vi "EC_Applied_Motion_SXSYSZ_20170419A_3chNoBK_20190710.vi"() -> ()   [LabVIEW 2015]
uses:
  <vilib>/Instr/_visa.llb/VISA Configure Serial Port (Instr).vi
  <userlib>/caLab/Private/Put_DBL_PV.vi
  <userlib>/caLab/Private/Get_PV-1D.vi
  <userlib>/caLab/Private/Put_I32-1D_PV-1D.vi
  <userlib>/caLab/Private/Put_DBL-1D_PV-1D.vi
  <vilib>/Utility/file.llb/Write To Spreadsheet File (I64).vi
  <vilib>/Utility/file.llb/Read From Spreadsheet File (I64).vi
panel:
  out "Io":dbl
  out "APX:MZ_CHK":bool[](array[boolean])
  out "x .and. y?":bool
  out "element 7":u8
  out "Busy":bool
  out "element 6":bool
  out "element 5":bool
  out "element 4":bool
  out "element 3":bool
  out "element 2":bool
  out "element":bool
  out "status":u32
  in  "Local":bool=TRUE
  out "Move 5Z REQ":bool
  in  "Jog Z- CNTL":bool
  in  "Jog Z+ CNTL":bool
  in  "Jog Y- CNTL":bool
  in  "Jog Y+ CNTL":bool
  in  "Jog X- CNTL":bool
  in  "Jog X+ CNTL":bool
  out "APX:FZ_DOWN":u8
  out "APX:FZ_UP":u8
  out "APX:FY_DOWN":u8
  out "APX:FY_UP":u8
  out "APX:FX_DOWN":u8
  out "APX:FX_UP":u8
  out "FZ Jog Counts In Range?":bool
  out "FY Jog Counts In Range?":bool
  out "FX Jog Counts In Range?":bool
  in  "APX:MZ_CHK local":bool=TRUE
  out "Isolated from GND?":bool
  in  "Crash Override":bool
  out "Dev1 AI1":dbl
  in  "APX:FZabs":dbl
  in  "Move 5Z":bool
  out "APX:FZ_DOWN":bool
  out "APX:FX_DOWN":bool
  out "APX:FY_DOWN":bool
  out "Z Velocity MV mm/sec":dbl format="%.3f"
  out "Z Position MV mm":dbl=0.09994900000000001 format="%#_3g"
  out "Y Velocity MV mm/sec":dbl format="%.3f"
  out "Y Position MV mm":dbl=0.049996453999999996 format="%#_3g"
  out "X Velocity MV mm/sec":dbl format="%.3f"
  out "X Position MV mm":dbl=0.1000034915 format="%#_3g"
  in  "stop":bool
  in  "Tab Control 3":enum32{"Status", "Reset", "Error"}(tab)
  out "Y in Range":bool
  out "Y in Motion":bool
  out "X  in Range":bool
  out "X  in Motion":bool
  out "Z in Range":bool
  out "Z in Motion":bool
  out "X Ready":bool
  out "Y Ready":bool
  out "Z Ready":bool
  in  "Reset Y Position mm":dbl
  out "Reset Y Motor Steps":i32
  in  "Reset X Position mm":dbl
  out "Reset X Motor Steps":i32
  in  "Reset Z Position mm":dbl
  out "Reset Z Motor Steps":i32
  in  "Reset":bool
  out "error out":errorcluster
  in  "Tab Control":enum32{"mm", "Jog", "step", "info"}(tab)
  in  "APX:FXstep":dbl=0.1 min=0.1 max=0.2
  in  "FX Velocity SP mm/sec":dbl=0.010583500000000001
  in  "APX:FYstep":dbl=0.05 min=0.01 max=0.1
  in  "FY Velocity SP mm/sec":dbl=0.010583500000000001
  in  "APX:Fzstep":dbl=0.05 min=0.05 max=0.2
  in  "FZ Velocity SP mm/sec":dbl=0.0635
  in  "Z Jog Set":bool
  in  "Y Jog Set":bool
  in  "X Jog Set":bool
  in  "Reset Jog counts":bool
  in  "FZ Jog counts":i8
  in  "FY Jog counts":i8
  in  "FX Jog counts":i8
  out "FX Jog upper limit":dbl=40.0
  out "FX Jog lower limit":dbl=-40.0
  out "FY Jog lower limit":dbl=-15.0
  out "FY jog upper limit":dbl=15.0
  out "FZ jog upper limit":dbl=40.0
  out "FZ Jog lower limit":dbl=-40.0
  in  "X Velocity SP step/sec":i32 min=1 max=1000
  in  "Y Velocity SP step/sec":i32 min=1 max=1000
  in  "Z Velocity SP step/sec":i32 min=1 max=500
  in  "Y Step SP":i32=-20000 min=-800000 max=800000 step=500
  in  "X Step SP":i32=-20000 min=-750000 max=750000 step=500
  in  "Z Step SP":i32=-20000 min=-10240000 max=10240000 step=500
  out "X Step PV":i32 max=2000
  out "Y Step PV":i32 max=2000
  out "Z Step PV":i32 max=2000
  out "R Step PV":i32 max=2000
  out "X Run Current %":i32
  out "X Holding Current %":i32
  out "X velocity PV step/sec":i32
  out "X steps/rev":u32
  out "X mm/rev":dbl
  out "X offset mm":dbl
  out "X MINPOS":i32=-94296
  out "X MAXPOS":i32=-34296
  out "X COM PORT":refnum<visa-resource-name>="COM5"
  out "Y COM PORT":refnum<visa-resource-name>="COM5"
  out "Z COM PORT":refnum<visa-resource-name>="COM5"
  out "Y velocity PV step/sec":i32
  out "Y Run Current %":i32
  out "Y Holding Current %":i32
  out "Y MAXPOS":i32=-34296
  out "Y MINPOS":i32=-94296
  out "Y steps/rev":u32
  out "Y mm/rev":dbl
  out "Y offset mm":dbl
  out "Z  velocity PV step/sec":i32
  out "Z Run Current %":i32
  out "Z Holding Current %":i32
  out "Z MAXPOS":i32=-34296
  out "Z MINPOS":i32=-94296
  out "Z steps/rev":u32
  out "Z mm/rev":dbl
  out "Z offset mm":dbl
  out "APX:FZ_UP":bool
  out "Z Position mm PV":dbl format="%.3f"
  out "X Position mm PV":dbl format="%.3g"
  out "APX:FX_UP":bool
  out "Y Position mm PV":dbl format="%.3g"
  in  "Stop":bool
  out "APX:FY_UP":bool
  # "APX:FY"
  # "APX:FinePos"
  # "APX:FZ"
  # "x-ray"
  # "v20220620"
  # "APX:FX"
  # "SPEAR"
  # "Stage"
  # "Velovity"
  # "Jog step"
  # "Pos"
  # "sample to SSRL"
  # "FX"
  # "FY"
  # "FZ"
  # "These have to be positive"
  # "lim"
  # "connected"
  # "moving"
  # "R,L = green"
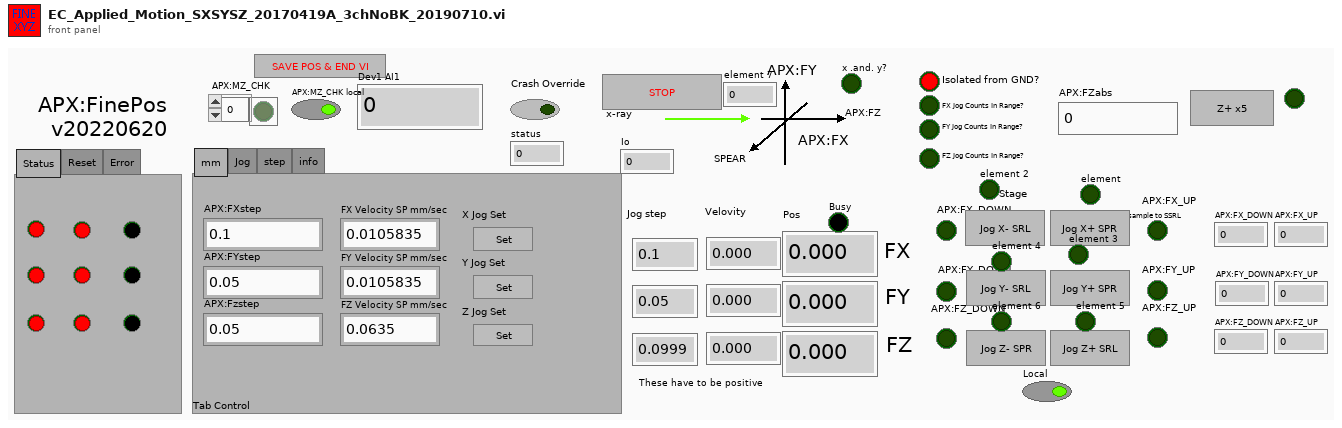
[diagram p1: front panel]
types:
  T1 = cluster{"first row[0]":i64, "first row[1]":i64, "first row[2]":i64, "first row[3]":i64, "first row[4]":i64, "first row[5]":i64, "first row[6]":i64, "first row[7]":i64, "first row[8]":i64}
  T2 = enum16{"Power-up Signature", "Accel Rate", "Accel Max", "Bit Rate", "Buffer Status", "Change Current", "Commence Jogging", "Change Jog Speed", "Continue", "Define Address", "Distance for FC,FM,FO,FY", "Decel Rate", "Distance or Position", "Define Limits", "Encoder Deadband", "Encoder Function", "Encoder Position", "Encoder Ratio", "Feed to Length with Speed Change", "Feed to Length", "Feed to Sensor with Mask Dist", "Feed to Length & Set Output", "Feed to Position", "Feed to Sensor", "Feed to Sensor w/safety", "Follow Handwheel", "Immediate Distance?", "Immediate Encoder?", "Immediate Low Output", "Immediate High Output", "Immediate Position?", "Input Status?", "Jog Accel/Decel", "Jog Disable", "Jog Enable", "Jog Speed", "Motor Disable", "Motor Enable", "Microstep Resolution", "Power up Current", "Power up Mode", "Pause", "Request Status", "Revision Level?", "Seek Home", "Stop Jogging", "Stop & Kill Buffer", "Set Output", "Set ABS Position", "Send String", "Stop", "Velocity for Speed Change", "Velocity Setting", "Wait for Input", "Wait Time"}
  T3 = enum8{"Enabled", "Disabled", "Disabled and Grayed Out"}
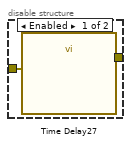
[diagram p7: hidden frame]
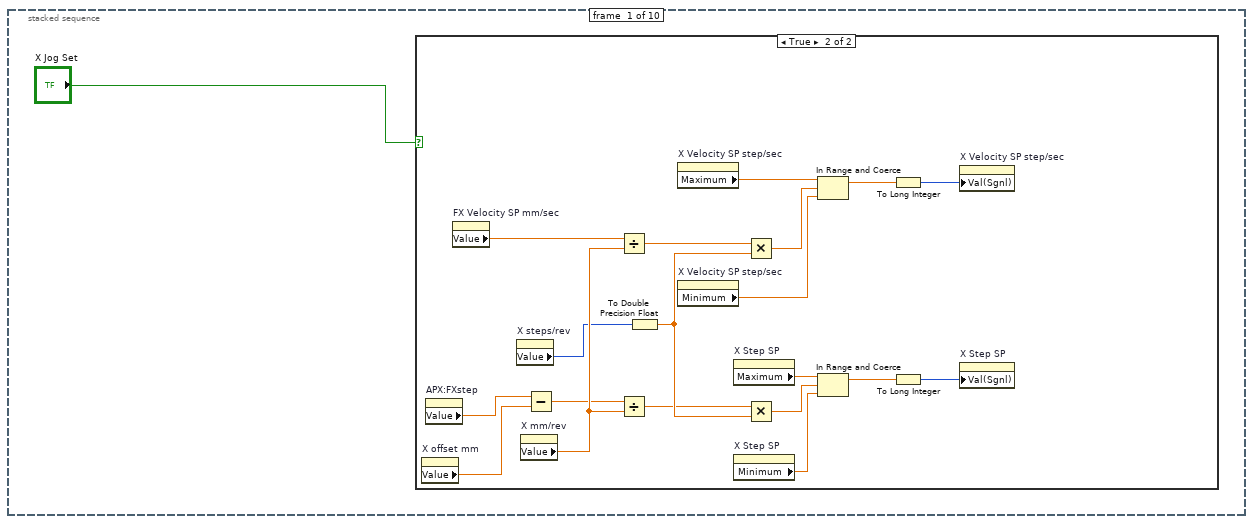
[diagram p9: hidden frame]
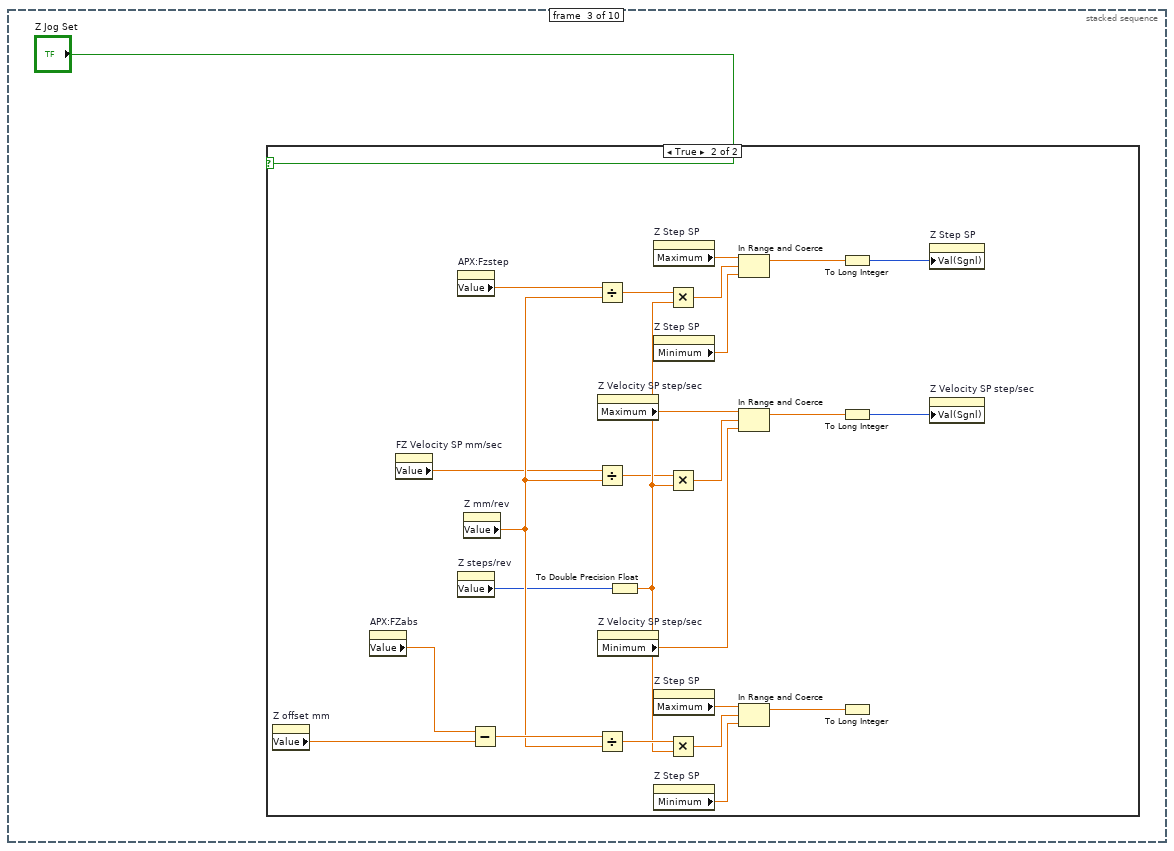
[diagram p12: hidden frame]
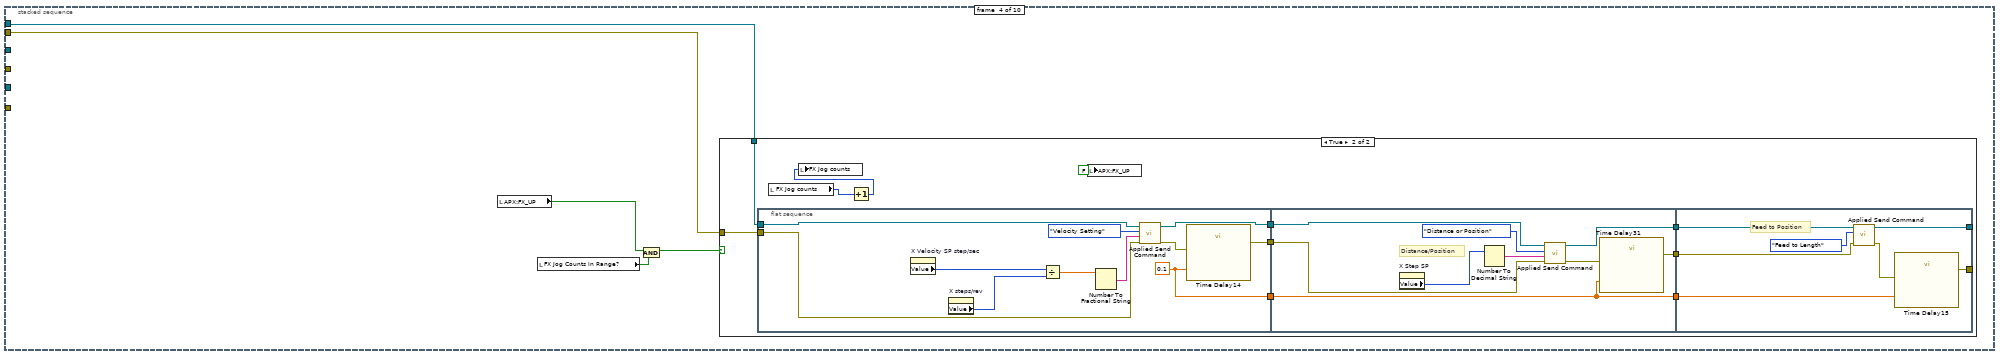
[diagram p14: hidden frame]
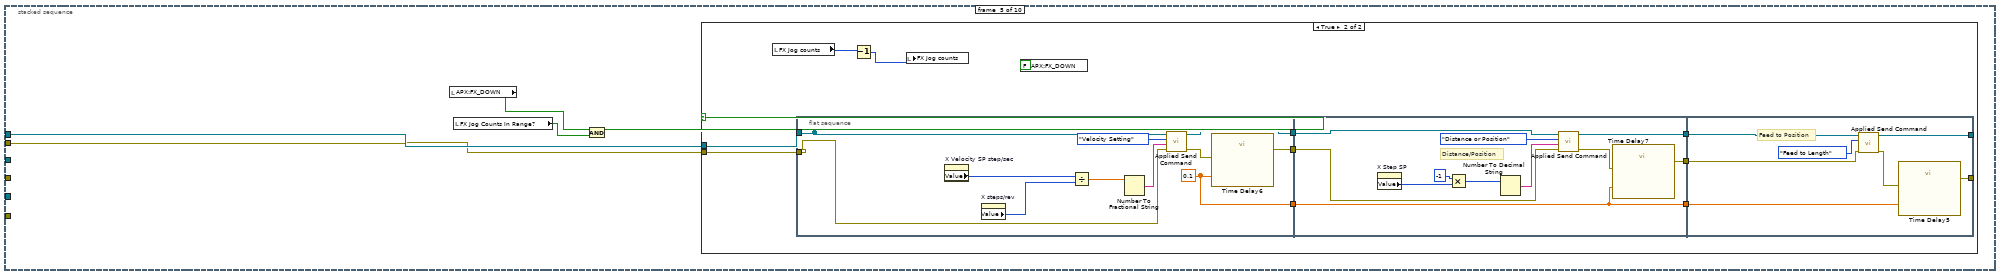
[diagram p16: hidden frame]
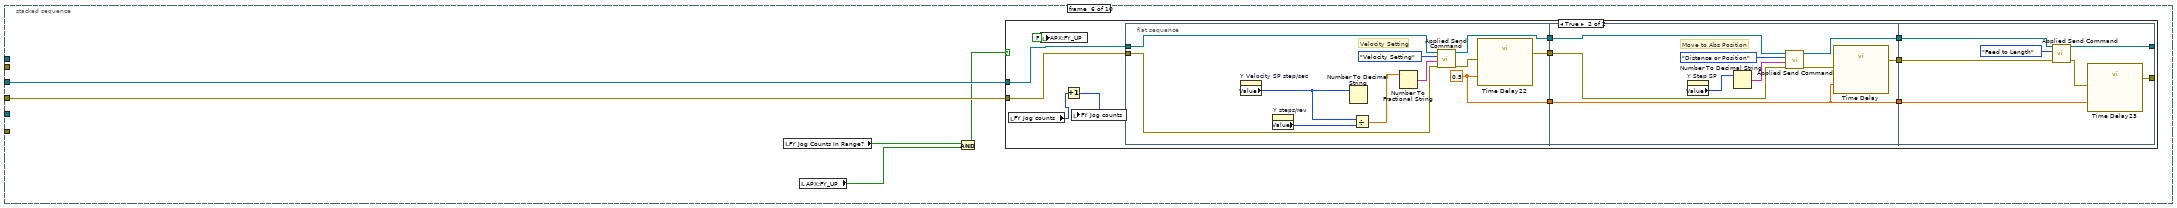
[diagram p18: hidden frame]
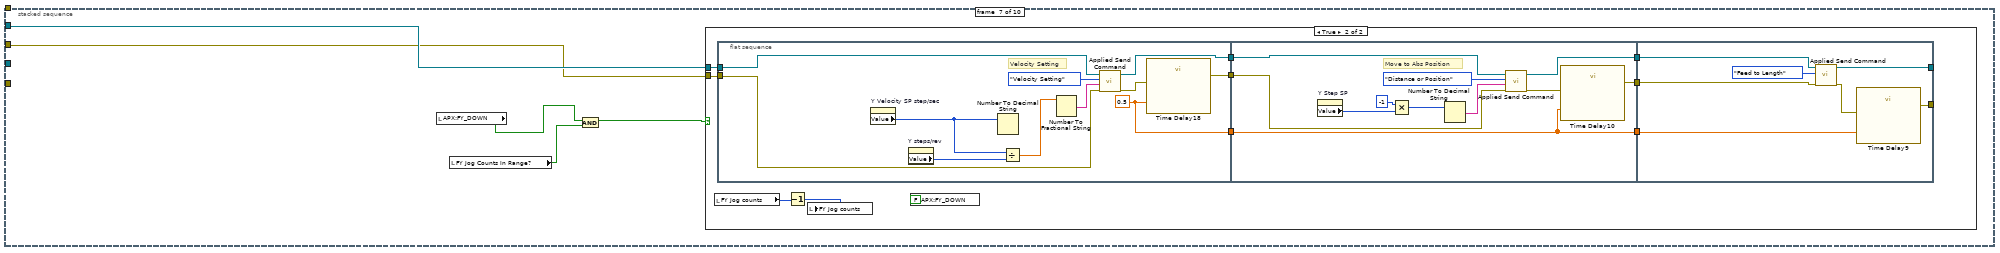
[diagram p20: hidden frame]
diagram:
  n1 = disable-structure shown="Disabled" {
    frame Disabled {
      (unwired) FALSE
      n2 = flat-sequence {
        frame #0 {
        }
        frame #1 {
          n3 = call-poly <vilib>:"Read From Spreadsheet File.vi"("file path (dialog if empty)"=path "S:/SSE/SCL2/POS.TXT") -> ("first row"=w43:i64[])  [unwired: 6 in, 4 out]
          n4 = Array To Cluster(array=w43) -> (cluster=w44:T1)
          n5 = Unbundle(w44) -> ("first row[0]"=w46:i64, "first row[1]"=w47:i64, "first row[2]"=w48:i64)  [unwired: 6 out]
          n6 = property on="Reset X Motor Steps" class="DigNum (strict)"("Val(Sgnl)"=w46) -> ()  [unwired: 2 in, 2 out]
          n7 = property on="Reset Y Motor Steps" class="DigNum (strict)"("Val(Sgnl)"=w47) -> ()  [unwired: 2 in, 2 out]
          n8 = property on="Reset Z Motor Steps" class="DigNum (strict)"("Val(Sgnl)"=w48) -> ()  [unwired: 2 in, 2 out]
        }
      }
    }
    frame Enabled {
    }
  }
  n9 = flat-sequence {
    tunnel: [w65] -> w18
    tunnel: [w64] -> w17
    tunnel: w18 -> [w82]
    tunnel: w17 -> [w81]
    tunnel: [w80] -> w16
    tunnel: [w79] -> w15
    tunnel: [w86] -> w40
    tunnel: w16 -> [w94]
    tunnel: w15 -> [w93]
    tunnel: [w87] -> w14
    tunnel: w40 -> [w108]
    tunnel: [w107] -> w34
    tunnel: [w105] -> w33
    tunnel: [w110] -> w32
    tunnel: w14 -> [w109]
    tunnel: [w116] -> w38
    tunnel: [w117] -> w39
    tunnel: w34 -> [w117]
    tunnel: w33 -> [w116]
    tunnel: w32 -> [w115]
    frame #0 {
      "X Run Current %" <- 100 ("Run Current %")
      "X Holding Current %" <- 50 ("Holding Current %")
    }
    frame #1 {
      w51 = T3."Enabled" ("Disabled")
      n10 = property on="APX:FX_UP" class="Bool"("DisabledEnum"=w51) -> ()  [unwired: 2 in, 2 out]
      n11 = property on="APX:FX_DOWN" class="Bool"("DisabledEnum"=w51) -> ()  [unwired: 2 in, 2 out]
      n12 = property on="APX:FY_UP" class="Bool"("DisabledEnum"=w51) -> ()  [unwired: 2 in, 2 out]
      n13 = property on="APX:FZ_UP" class="Bool"("DisabledEnum"=w51) -> ()  [unwired: 2 in, 2 out]
      n14 = property on="APX:FY_DOWN" class="Bool"("DisabledEnum"=w51) -> ()  [unwired: 2 in, 2 out]
      n15 = property on="APX:FZ_DOWN" class="Bool"("DisabledEnum"=w51) -> ()  [unwired: 2 in, 2 out]
    }
    frame #2 {
      w54 = 0.21167 ("MM/rev")
      w57 = u32 20000 ("step/rev")
      w52 = 1000 ("Value (Signaling)")
      (unwired) 0.01 ("Value (Signaling)")
      n16 = property on="X Velocity SP step/sec" class="DigNum (strict)"("Minimum"=1.0 ("Data Entry Limits:Minimum")) -> ()  [unwired: 2 in, 2 out]
      n17 = property on="X Velocity SP step/sec" class="DigNum (strict)"("Val(Sgnl)"=w52) -> ()  [unwired: 2 in, 2 out]
      n18 = To Double Precision Float(number=w57) -> (double precision float=w56:dbl)
      n19 = To Double Precision Float(number=w52) -> (double precision float=w58:dbl)
      n20 = property on="X Velocity SP step/sec" class="DigNum (strict)"("Maximum"=w58) -> ()  [unwired: 2 in, 2 out]
      n21 = Divide(x=w58, y=w56) -> (x/y=w53:dbl)
      n22 = Multiply(x=w53, y=w54) -> (x*y=w55:dbl)
      n23 = property on="FX Velocity SP mm/sec" class="DigNum (strict)"("Val(Sgnl)"=w55) -> ()  [unwired: 2 in, 2 out]
      "X steps/rev" <- w57
      "X mm/rev" <- w54
    }
    frame #3 {
      w63 = -750000 ("lower limit")
      w62 = 750000 ("upper limit")
      n24 = local write "X Step SP"(9449 ("X Step SP")) -> ()
      n25 = property on="X Step SP" class="DigNum (strict)"("Maximum"=w62) -> ()  [unwired: 2 in, 2 out]
      n26 = property on="X Step SP" class="DigNum (strict)"("Minimum"=w63) -> ()  [unwired: 2 in, 2 out]
      "X offset mm" <- 0.0 ("offset")
      "X MAXPOS" <- w62
      "X MINPOS" <- w63
    }
    frame #4 {
      w72 = refnum<visa-resource-name> "COM21" ("COM PORT")
      w70 = u16 0 items=["None", "XON/XOFF", "RTS/CTS", "XON/XOFF & RTS/CTS", "DTR/DSR", "XON/XOFF & DTR/DSR"] ("flow control (0:none)")
      w69 = u16 10 items=["1.0"=10, "1.5"=15, "2.0"=20] ("stop bits (10: 1 bit)")
      # "Stop bits"
      n27 = call-poly "VISA Configure Serial Port"("VISA resource name"=w72, "timeout (10sec)"=u32 10000, "baud rate (9600)"=u32 9600, "data bits (8)"=u16 8, "parity (0:none)"=enum16{"None", "Odd", "Even", "Mark", "Space"}."None", "stop bits (10: 1 bit)"=w69, "flow control (0:none)"=w70) -> ("VISA resource name out"=w65:refnum<visa-resource-name>, "error out"=w64:errorcluster)  [unwired: 7 in]
      "X COM PORT" <- w72
    }
    frame #5 {
      n28 = property on="X Run Current" class="DigNum (strict)"() -> ("Value"=w77:i32)  [unwired: 2 in, 2 out]
      n29 = Divide(x=w77, y=100) -> (x/y=w74:dbl)
      n30 = Multiply(x=3.5 ("y"), y=w74) -> (x*y=w76:dbl)
      n31 = Number To Fractional String(number=w76) -> (F-format string=w78:string)  [unwired: 3 in]
      n32 = call "Applied Send Command.vi"("error in (no error)"=w81, "Extra"=w78, "Command"=T2."Change Current", "VISA resource name"=w82) -> ("error out"=w80:errorcluster, "VISA resource name out"=w79:refnum<visa-resource-name>)  [unwired: 3 in, 1 out]
    }
    frame #6 {
      # "VELOCITY"
      n33 = property on="X Velocity SP step/sec" class="DigNum (strict)"() -> ("Value"=w90:i32)  [unwired: 2 in, 2 out]
      n34 = property on="X steps/rev" class="DigNum (strict)"() -> ("Value"=w89:u32)  [unwired: 2 in, 2 out]
      n35 = Divide(x=w90, y=w89) -> (x/y=w88:dbl)
      n36 = Absolute Value(x=w88) -> (abs(x)=w84:dbl)
      n37 = Number To Fractional String(number=w84) -> (F-format string=w95:string)  [unwired: 3 in]
      n38 = call "Applied Send Command.vi"("error in (no error)"=w94, "Extra"=w95, "Command"=T2."Velocity Setting", "VISA resource name"=w93) -> ("error out"=w96:errorcluster, "VISA resource name out"=w103:refnum<visa-resource-name>)  [unwired: 3 in, 1 out]
      n39 = call "Time Delay30"("error in (no error)"=w96, "Delay Time (s)"=0.1) -> ("error out"=w101:errorcluster)  [unwired: 9 in]
      n40 = call "Applied Send Command.vi"("error in (no error)"=w101, "Extra"="", "Command"=T2."Velocity Setting", "VISA resource name"=w103) -> ("error out"=w86:errorcluster, "read buffer"=w99:string, "VISA resource name out"=w87:refnum<visa-resource-name>)  [unwired: 3 in]
      n41 = Fract/Exp String To Number(string=w99, offset=3) -> (number=w92:dbl)  [unwired: 2 in, 1 out]
      n42 = Multiply(x=w92, y=w89) -> (x*y=w91:dbl)
      n43 = property on="X velocity PV step/sec" class="DigNum (strict)"("Val(Sgnl)"=w91) -> ()  [unwired: 2 in, 2 out]
    }
    frame #7 {
      # "GET CURRENT POSITION"
      n44 = call "Applied Send Command.vi"("error in (no error)"=w108, "Extra"="", "Command"=T2."Immediate Position?", "VISA resource name"=w109) -> ("error out"=w106:errorcluster, "read buffer"=w112:string, "VISA resource name out"=w107:refnum<visa-resource-name>)  [unwired: 3 in]
      n45 = call "Time Delay13"("error in (no error)"=w106, "Delay Time (s)"=0.1) -> ("error out"=w105:errorcluster)  [unwired: 9 in]
      n46 = Hexadecimal String To Number(string=w112, offset=3) -> (number=w110:u32)  [unwired: 1 in, 1 out]
    }
    frame #8 {
      n47 = disable-structure shown="Disabled" {
        disable-tunnel: w115 -> [w118 _]
        frame Disabled {
          n48 = property on="X Step SP" class="DigNum (strict)"("Val(Sgnl)"=w118) -> ()  [unwired: 2 in, 2 out]
          n49 = property on="X Step SP" class="DigNum (strict)"() -> ("Maximum"=w121:dbl)  [unwired: 2 in, 2 out]
          n50 = property on="X Step SP" class="DigNum (strict)"() -> ("Minimum"=w120:dbl)  [unwired: 2 in, 2 out]
          n51 = In Range and Coerce(upper limit=w121, x=w118, lower limit=w120) -> (In Range?=w119:bool)  [unwired: 1 out]
          n52 = property on="X  in Range" class="Bool (strict)"("Val(Sgnl)"=w119) -> ()  [unwired: 2 in, 2 out]
        }
        frame Enabled {
        }
      }
    }
  }
  n53 = flat-sequence {
    tunnel: [w137] -> w5
    tunnel: [w136] -> w4
    tunnel: w5 -> [w151]
    tunnel: w4 -> [w150]
    tunnel: [w149] -> w3
    tunnel: [w148] -> w2
    tunnel: [w160] -> w31
    tunnel: [w159] -> w30
    tunnel: w3 -> [w162]
    tunnel: w2 -> [w161]
    tunnel: w31 -> [w177]
    tunnel: w30 -> [w176]
    tunnel: [w178] -> w29
    tunnel: [w179] -> w28
    tunnel: [w180] -> w1
    tunnel: [w190] -> w26
    tunnel: [w191] -> w27
    tunnel: w29 -> [w191]
    tunnel: w28 -> [w190]
    tunnel: w1 -> [w189]
    frame #0 {
      "Z Run Current %" <- 100 ("Z Run Current %")
      "Z Holding Current %" <- 50 ("Z Holding Current %")
    }
    frame #1 {
    }
    frame #2 {
      (unwired) 0.05 ("Value (Signaling)")
      w126 = 2.54 ("Z mm/rev")
      w125 = u32 20000 ("step/rev")
      w127 = 500 ("Value (Signaling)")
      n54 = property on="Z Velocity SP step/sec" class="DigNum (strict)"("Minimum"=1.0 ("Data Entry Limits:Minimum")) -> ()  [unwired: 2 in, 2 out]
      n55 = property on="Z Velocity SP step/sec" class="DigNum (strict)"("Val(Sgnl)"=w127) -> ()  [unwired: 2 in, 2 out]
      n56 = To Double Precision Float(number=w125) -> (double precision float=w130:dbl)
      n57 = To Double Precision Float(number=w127) -> (double precision float=w131:dbl)
      n58 = property on="Z Velocity SP step/sec" class="DigNum (strict)"("Maximum"=w131) -> ()  [unwired: 2 in, 2 out]
      n59 = Divide(x=w131, y=w130) -> (x/y=w128:dbl)
      n60 = Multiply(x=w128, y=w126) -> (x*y=w129:dbl)
      n61 = property on="FZ Velocity SP mm/sec" class="DigNum (strict)"("Val(Sgnl)"=w129) -> ()  [unwired: 2 in, 2 out]
      "Z mm/rev" <- w126
      "Z steps/rev" <- w125
    }
    frame #3 {
      w134 = -10240000 ("lower limit")
      w133 = 10240000 ("upper limit")
      n62 = property on="Z Step SP" class="DigNum (strict)"("Minimum"=w134) -> ()  [unwired: 2 in, 2 out]
      n63 = local write "Z Step SP"(394 ("Z Step SP")) -> ()
      n64 = property on="Z Step SP" class="DigNum (strict)"("Maximum"=w133) -> ()  [unwired: 2 in, 2 out]
      "Z offset mm" <- 0.0 ("Z offset mm")
      "Z MINPOS" <- w134
      "Z MAXPOS" <- w133
    }
    frame #4 {
      w144 = refnum<visa-resource-name> "COM23" ("COM PORT")
      w142 = u16 0 items=["None", "XON/XOFF", "RTS/CTS", "XON/XOFF & RTS/CTS", "DTR/DSR", "XON/XOFF & DTR/DSR"] ("flow control (0:none)")
      w141 = u16 10 items=["1.0"=10, "1.5"=15, "2.0"=20] ("stop bits (10: 1 bit)")
      # "Stop bits"
      n65 = call-poly "VISA Configure Serial Port"("VISA resource name"=w144, "timeout (10sec)"=u32 10000, "baud rate (9600)"=u32 9600, "data bits (8)"=u16 8, "parity (0:none)"=enum16{"None", "Odd", "Even", "Mark", "Space"}."None", "stop bits (10: 1 bit)"=w141, "flow control (0:none)"=w142) -> ("VISA resource name out"=w137:refnum<visa-resource-name>, "error out"=w136:errorcluster)  [unwired: 7 in]
      "Z COM PORT" <- w144
    }
    frame #5 {
      # "Run Current %"
      n66 = property on="Z Run Current %" class="DigNum (strict)"() -> ("Value"=w152:i32)  [unwired: 2 in, 2 out]
      n67 = Divide(x=w152, y=100) -> (x/y=w153:dbl)
      n68 = Multiply(x=w153, y=3.5) -> (x*y=w147:dbl)
      n69 = Number To Fractional String(number=w147) -> (F-format string=w154:string)  [unwired: 3 in]
      n70 = call "Applied Send Command.vi"("error in (no error)"=w150, "Extra"=w154, "Command"=T2."Change Current", "VISA resource name"=w151) -> ("error out"=w148:errorcluster, "VISA resource name out"=w149:refnum<visa-resource-name>)  [unwired: 3 in, 1 out]
    }
    frame #6 {
      # "VELOCITY"
      n71 = property on="Z Velocity SP step/sec" class="DigNum (strict)"() -> ("Value"=w157:i32)  [unwired: 2 in, 2 out]
      n72 = property on="Z steps/rev" class="DigNum (strict)"() -> ("Value"=w158:u32)  [unwired: 2 in, 2 out]
      n73 = Divide(x=w157, y=w158) -> (x/y=w165:dbl)
      n74 = Absolute Value(x=w165) -> (abs(x)=w156:dbl)
      n75 = Number To Fractional String(number=w156) -> (F-format string=w167:string)  [unwired: 3 in]
      n76 = call "Applied Send Command.vi"("error in (no error)"=w161, "Extra"=w167, "Command"=T2."Velocity Setting", "VISA resource name"=w162) -> ("error out"=w168:errorcluster, "VISA resource name out"=w175:refnum<visa-resource-name>)  [unwired: 3 in, 1 out]
      n77 = call "Time Delay2"("error in (no error)"=w168, "Delay Time (s)"=0.1) -> ("error out"=w173:errorcluster)  [unwired: 9 in]
      n78 = call "Applied Send Command.vi"("error in (no error)"=w173, "Extra"="", "Command"=T2."Velocity Setting", "VISA resource name"=w175) -> ("error out"=w159:errorcluster, "read buffer"=w171:string, "VISA resource name out"=w160:refnum<visa-resource-name>)  [unwired: 3 in]
      n79 = Fract/Exp String To Number(string=w171, offset=3) -> (number=w166:dbl)  [unwired: 2 in, 1 out]
      n80 = Multiply(x=w166, y=w158) -> (x*y=w163:dbl)
      n81 = property on="Z  velocity PV step/sec" class="DigNum (strict)"("Val(Sgnl)"=w163) -> ()  [unwired: 2 in, 2 out]
    }
    frame #7 {
      # "GET CURRENT POSITION"
      n82 = call "Applied Send Command.vi"("error in (no error)"=w176, "Extra"="", "Command"=T2."Immediate Position?", "VISA resource name"=w177) -> ("error out"=w182:errorcluster, "read buffer"=w184:string, "VISA resource name out"=w178:refnum<visa-resource-name>)  [unwired: 3 in]
      n83 = call "Time Delay8"("error in (no error)"=w182, "Delay Time (s)"=0.1) -> ("error out"=w179:errorcluster)  [unwired: 9 in]
      n84 = Hexadecimal String To Number(string=w184, offset=3) -> (number=w180:u32)  [unwired: 1 in, 1 out]
    }
    frame #8 {
      n85 = disable-structure shown="Disabled" {
        disable-tunnel: w189 -> [w194 _]
        frame Disabled {
          n86 = property on="Z Step SP" class="DigNum (strict)"("Val(Sgnl)"=w194) -> ()  [unwired: 2 in, 2 out]
          n87 = property on="Z Step SP" class="DigNum (strict)"() -> ("Maximum"=w193:dbl)  [unwired: 2 in, 2 out]
          n88 = property on="Z Step SP" class="DigNum (strict)"() -> ("Minimum"=w192:dbl)  [unwired: 2 in, 2 out]
          n89 = In Range and Coerce(upper limit=w193, x=w194, lower limit=w192) -> (In Range?=w195:bool)  [unwired: 1 out]
          n90 = property on="Z in Range" class="Bool (strict)"("Val(Sgnl)"=w195) -> ()  [unwired: 2 in, 2 out]
        }
        frame Enabled {
        }
      }
      n91 = property on="Z Position MV mm" class="DigNum (strict)"("Val(Sgnl)"=0.05 ("Value (Signaling)")) -> ()  [unwired: 2 in, 2 out]
      n92 = property on="X Position MV mm" class="DigNum (strict)"("Val(Sgnl)"=0.1 ("Value (Signaling)")) -> ()  [unwired: 2 in, 2 out]
    }
  }
  n93 = flat-sequence {
    tunnel: [w211] -> w13
    tunnel: [w210] -> w12
    tunnel: w13 -> [w225]
    tunnel: w12 -> [w224]
    tunnel: [w223] -> w11
    tunnel: [w222] -> w10
    tunnel: w11 -> [w234]
    tunnel: w10 -> [w233]
    tunnel: [w232] -> w9
    tunnel: [w231] -> w8
    tunnel: [w251] -> w35
    tunnel: w9 -> [w254]
    tunnel: w8 -> [w253]
    tunnel: [w252] -> w7
    tunnel: [w250] -> w6
    tunnel: [w262] -> w41
    tunnel: [w264] -> w42
    tunnel: w35 -> [w262]
    tunnel: w7 -> [w264]
    tunnel: w6 -> [w263]
    frame #0 {
      "Y Run Current %" <- 100 ("Run Current %")
      "Y Holding Current %" <- 50 ("Holding Current %")
    }
    frame #1 {
    }
    frame #2 {
      w200 = 0.21167 ("MM/rev")
      w203 = u32 20000 ("step/rev")
      w198 = 1000 ("Value (Signaling)")
      (unwired) 0.01 ("Value (Signaling)")
      n94 = property on="Y Velocity SP step/sec" class="DigNum (strict)"("Minimum"=1.0 ("Data Entry Limits:Minimum")) -> ()  [unwired: 2 in, 2 out]
      n95 = property on="Y Velocity SP step/sec" class="DigNum (strict)"("Val(Sgnl)"=w198) -> ()  [unwired: 2 in, 2 out]
      n96 = To Double Precision Float(number=w203) -> (double precision float=w202:dbl)
      n97 = To Double Precision Float(number=w198) -> (double precision float=w204:dbl)
      n98 = property on="Y Velocity SP step/sec" class="DigNum (strict)"("Maximum"=w204) -> ()  [unwired: 2 in, 2 out]
      n99 = Divide(x=w204, y=w202) -> (x/y=w199:dbl)
      n100 = Multiply(x=w199, y=w200) -> (x*y=w201:dbl)
      n101 = property on="FY Velocity SP mm/sec" class="DigNum (strict)"("Val(Sgnl)"=w201) -> ()  [unwired: 2 in, 2 out]
      "Y steps/rev" <- w203
      "Y mm/rev" <- w200
    }
    frame #3 {
      w208 = -800000 ("lower limit")
      w209 = 800000 ("upper limit")
      n102 = local write "Y Step SP"(4724 ("Y Step SP")) -> ()
      n103 = property on="Y Step SP" class="DigNum (strict)"("Maximum"=w209) -> ()  [unwired: 2 in, 2 out]
      n104 = property on="Y Step SP" class="DigNum (strict)"("Minimum"=w208) -> ()  [unwired: 2 in, 2 out]
      "Y MAXPOS" <- w209
      "Y MINPOS" <- w208
      "Y offset mm" <- 0.0 ("offset")
    }
    frame #4 {
      w218 = refnum<visa-resource-name> "COM22" ("COM PORT")
      w216 = u16 0 items=["None", "XON/XOFF", "RTS/CTS", "XON/XOFF & RTS/CTS", "DTR/DSR", "XON/XOFF & DTR/DSR"] ("flow control (0:none)")
      w215 = u16 10 items=["1.0"=10, "1.5"=15, "2.0"=20] ("stop bits (10: 1 bit)")
      # "Stop bits"
      n105 = call-poly "VISA Configure Serial Port"("VISA resource name"=w218, "timeout (10sec)"=u32 10000, "baud rate (9600)"=u32 9600, "data bits (8)"=u16 8, "parity (0:none)"=enum16{"None", "Odd", "Even", "Mark", "Space"}."None", "stop bits (10: 1 bit)"=w215, "flow control (0:none)"=w216) -> ("VISA resource name out"=w211:refnum<visa-resource-name>, "error out"=w210:errorcluster)  [unwired: 7 in]
      "Y COM PORT" <- w218
    }
    frame #5 {
      n106 = property on="Y Run Current %" class="DigNum (strict)"() -> ("Value"=w226:i32)  [unwired: 2 in, 2 out]
      n107 = Divide(x=w226, y=100) -> (x/y=w227:dbl)
      n108 = Multiply(x=w227, y=3.5) -> (x*y=w221:dbl)
      n109 = Number To Fractional String(number=w221) -> (F-format string=w228:string)  [unwired: 3 in]
      n110 = call "Applied Send Command.vi"("error in (no error)"=w224, "Extra"=w228, "Command"=T2."Change Current", "VISA resource name"=w225) -> ("error out"=w222:errorcluster, "VISA resource name out"=w223:refnum<visa-resource-name>)  [unwired: 3 in, 1 out]
    }
    frame #6 {
      # "VELOCITY"
      n111 = property on="Y Velocity SP step/sec" class="DigNum (strict)"() -> ("Value"=w235:i32)  [unwired: 2 in, 2 out]
      n112 = property on="Y steps/rev" class="DigNum (strict)"() -> ("Value"=w238:u32)  [unwired: 2 in, 2 out]
      n113 = Divide(x=w235, y=w238) -> (x/y=w237:dbl)
      n114 = Absolute Value(x=w237) -> (abs(x)=w230:dbl)
      n115 = Number To Fractional String(number=w230) -> (F-format string=w241:string)  [unwired: 3 in]
      n116 = call "Applied Send Command.vi"("error in (no error)"=w233, "Extra"=w241, "Command"=T2."Velocity Setting", "VISA resource name"=w234) -> ("error out"=w242:errorcluster, "VISA resource name out"=w249:refnum<visa-resource-name>)  [unwired: 3 in, 1 out]
      n117 = call "Time Delay36"("error in (no error)"=w242, "Delay Time (s)"=0.1) -> ("error out"=w247:errorcluster)  [unwired: 9 in]
      n118 = call "Applied Send Command.vi"("error in (no error)"=w247, "Extra"="", "Command"=T2."Velocity Setting", "VISA resource name"=w249) -> ("error out"=w231:errorcluster, "read buffer"=w245:string, "VISA resource name out"=w232:refnum<visa-resource-name>)  [unwired: 3 in]
      n119 = Fract/Exp String To Number(string=w245, offset=3) -> (number=w240:dbl)  [unwired: 2 in, 1 out]
      n120 = Multiply(x=w240, y=w238) -> (x*y=w239:dbl)
      n121 = property on="Y velocity PV step/sec" class="DigNum (strict)"("Val(Sgnl)"=w239) -> ()  [unwired: 2 in, 2 out]
    }
    frame #7 {
      # "GET CURRENT POSITION"
      n122 = call "Applied Send Command.vi"("error in (no error)"=w253, "Extra"="", "Command"=T2."Immediate Position?", "VISA resource name"=w254) -> ("error out"=w256:errorcluster, "read buffer"=w258:string, "VISA resource name out"=w252:refnum<visa-resource-name>)  [unwired: 3 in]
      n123 = call "Time Delay37"("error in (no error)"=w256, "Delay Time (s)"=0.1) -> ("error out"=w251:errorcluster)  [unwired: 9 in]
      n124 = Hexadecimal String To Number(string=w258, offset=3) -> (number=w250:u32)  [unwired: 1 in, 1 out]
    }
    frame #8 {
      n125 = disable-structure shown="Disabled" {
        disable-tunnel: w263 -> [w267 _]
        frame Disabled {
          n126 = property on="Y Step SP" class="DigNum (strict)"("Val(Sgnl)"=w267) -> ()  [unwired: 2 in, 2 out]
          n127 = property on="Y Step SP" class="DigNum (strict)"() -> ("Maximum"=w266:dbl)  [unwired: 2 in, 2 out]
          n128 = property on="Y Step SP" class="DigNum (strict)"() -> ("Minimum"=w265:dbl)  [unwired: 2 in, 2 out]
          n129 = In Range and Coerce(upper limit=w266, x=w267, lower limit=w265) -> (In Range?=w268:bool)  [unwired: 1 out]
          n130 = property on="Y in Range" class="Bool (strict)"("Val(Sgnl)"=w268) -> ()  [unwired: 2 in, 2 out]
        }
        frame Enabled {
        }
      }
      n131 = property on="Y Position MV mm" class="DigNum (strict)"("Val(Sgnl)"=0.05 ("Value (Signaling)")) -> ()  [unwired: 2 in, 2 out]
    }
  }
  n132 = while {
    tunnel: w42 -> [w273]
    tunnel: w41 -> [w272]
    tunnel: [w285] -> w22
    tunnel: [w284] -> w23
    tunnel: w39 -> [w275]
    tunnel: w38 -> [w274]
    tunnel: [w282] -> w37
    tunnel: [w281] -> w36
    tunnel: w27 -> [w271]
    tunnel: w26 -> [w270]
    tunnel: [w280] -> w25
    tunnel: [w279] -> w24
    tunnel: [w278] -> _
    tunnel: [w277] -> _
    stop <- "stop" stop-if-true
    n133 = flat-sequence {
      frame #0 {
      }
      frame #1 {
      }
    }
    n134 = flat-sequence {
      frame #0 {
      }
      frame #1 {
      }
    }
    n135 = flat-sequence {
      frame #0 {
        n136 = local read "X Position mm PV"() -> (w292:dbl)
        n137 = local read "Z Position mm PV"() -> (w293:dbl)
        n138 = local read "Y Position mm PV"() -> (w291:dbl)
        n139 = Build Array(w292, w291, w293) -> (w286:dbl[])
        n140 = Build Array("APX:PiezeX", "APX:PiezeY", "APX:PiezeZ") -> (w287:string[])
        n141 = call-poly <userlib>:"CaLabPut.vi"("Values"=w286, "PV Names"=w287) -> ()  [unwired: 6 in, 4 out]
      }
    }
    n142 = flat-sequence {
      frame #0 {
        w297 = -40.0 ("lower limit")
        w296 = 40.0 ("upper limit")
        w301 = -15.0 ("lower limit")
        w300 = 15.0 ("upper limit")
        w305 = -40.0 ("lower limit")
        w304 = 40.0 ("upper limit")
        n143 = local read "FZ Jog counts"() -> (w295:i8)
        n144 = local read "FY Jog counts"() -> (w299:i8)
        n145 = local read "FX Jog counts"() -> (w303:i8)
        n146 = In Range and Coerce(upper limit=w304, x=w303, lower limit=w305) -> (In Range?=→"FX Jog Counts In Range?":bool)  [unwired: 1 out]
        n147 = In Range and Coerce(upper limit=w300, x=w299, lower limit=w301) -> (In Range?=→"FY Jog Counts In Range?":bool)  [unwired: 1 out]
        n148 = In Range and Coerce(upper limit=w296, x=w295, lower limit=w297) -> (In Range?=→"FZ Jog Counts In Range?":bool)  [unwired: 1 out]
        "FX Jog upper limit" <- w304
        "FX Jog lower limit" <- w305
        "FY jog upper limit" <- w300
        "FY Jog lower limit" <- w301
        "FZ jog upper limit" <- w296
        "FZ Jog lower limit" <- w297
      }
    }
    n149 = stacked-sequence {
      tunnel: w275 -> [_ _ _ w477 w520 _ _ _ _ _]
      tunnel: w274 -> [_ _ _ w476 w519 _ _ _ _ _]
      tunnel: w273 -> [_ _ _ _ _ w565 w608 _ _ _]
      tunnel: w272 -> [_ _ _ _ _ w564 w607 _ _ _]
      tunnel: w271 -> [_ _ _ _ _ _ _ w653 w696 w740]
      tunnel: w270 -> [_ _ _ _ _ _ _ w652 w695 w741]
      frame #0 {
        n150 = case shown="True" "X Jog Set" {
          frame False {
          }
          frame True {
            n151 = property on="X offset mm" class="DigNum (strict)"() -> ("Value"=w412:dbl)  [unwired: 2 in, 2 out]
            n152 = property on="APX:FXstep" class="DigNum (strict)"() -> ("Value"=w413:dbl)  [unwired: 2 in, 2 out]
            n153 = property on="FX Velocity SP mm/sec" class="DigNum (strict)"() -> ("Value"=w419:dbl)  [unwired: 2 in, 2 out]
            n154 = property on="X steps/rev" class="DigNum (strict)"() -> ("Value"=w410:u32)  [unwired: 2 in, 2 out]
            n155 = property on="X mm/rev" class="DigNum (strict)"() -> ("Value"=w426:dbl)  [unwired: 2 in, 2 out]
            n156 = Subtract(x=w413, y=w412) -> (x-y=w409:dbl)
            n157 = Divide(x=w419, y=w426) -> (x/y=w418:dbl)
            n158 = Divide(x=w409, y=w426) -> (x/y=w408:dbl)
            n159 = To Double Precision Float(number=w410) -> (double precision float=w425:dbl)
            n160 = property on="X Velocity SP step/sec" class="DigNum (strict)"() -> ("Maximum"=w423:dbl)  [unwired: 2 in, 2 out]
            n161 = property on="X Velocity SP step/sec" class="DigNum (strict)"() -> ("Minimum"=w424:dbl)  [unwired: 2 in, 2 out]
            n162 = property on="X Step SP" class="DigNum (strict)"() -> ("Maximum"=w416:dbl)  [unwired: 2 in, 2 out]
            n163 = property on="X Step SP" class="DigNum (strict)"() -> ("Minimum"=w417:dbl)  [unwired: 2 in, 2 out]
            n164 = Multiply(x=w418, y=w425) -> (x*y=w421:dbl)
            n165 = Multiply(x=w408, y=w425) -> (x*y=w414:dbl)
            n166 = In Range and Coerce(upper limit=w423, x=w421, lower limit=w424) -> (coerced(x)=w422:dbl)  [unwired: 1 out]
            n167 = In Range and Coerce(upper limit=w416, x=w414, lower limit=w417) -> (coerced(x)=w415:dbl)  [unwired: 1 out]
            n168 = To Long Integer(number=w422) -> (32bit integer=w420:i32)
            n169 = To Long Integer(number=w415) -> (32bit integer=w411:i32)
            n170 = property on="X Velocity SP step/sec" class="DigNum (strict)"("Val(Sgnl)"=w420) -> ()  [unwired: 2 in, 2 out]
            n171 = property on="X Step SP" class="DigNum (strict)"("Val(Sgnl)"=w411) -> ()  [unwired: 2 in, 2 out]
          }
        }
      }
      frame #1 {
        n172 = case shown="True" "Y Jog Set" {
          frame False {
          }
          frame True {
            n173 = property on="Y offset mm" class="DigNum (strict)"() -> ("Value"=w432:dbl)  [unwired: 2 in, 2 out]
            n174 = property on="APX:FYstep" class="DigNum (strict)"() -> ("Value"=w433:dbl)  [unwired: 2 in, 2 out]
            n175 = property on="FY Velocity SP mm/sec" class="DigNum (strict)"() -> ("Value"=w439:dbl)  [unwired: 2 in, 2 out]
            n176 = property on="Y steps/rev" class="DigNum (strict)"() -> ("Value"=w430:u32)  [unwired: 2 in, 2 out]
            n177 = property on="Y mm/rev" class="DigNum (strict)"() -> ("Value"=w446:dbl)  [unwired: 2 in, 2 out]
            n178 = Subtract(x=w433, y=w432) -> (x-y=w429:dbl)
            n179 = Divide(x=w439, y=w446) -> (x/y=w438:dbl)
            n180 = Divide(x=w429, y=w446) -> (x/y=w428:dbl)
            n181 = To Double Precision Float(number=w430) -> (double precision float=w445:dbl)
            n182 = property on="Y Velocity SP step/sec" class="DigNum (strict)"() -> ("Maximum"=w443:dbl)  [unwired: 2 in, 2 out]
            n183 = property on="Y Velocity SP step/sec" class="DigNum (strict)"() -> ("Minimum"=w444:dbl)  [unwired: 2 in, 2 out]
            n184 = property on="Y Step SP" class="DigNum (strict)"() -> ("Maximum"=w436:dbl)  [unwired: 2 in, 2 out]
            n185 = property on="Y Step SP" class="DigNum (strict)"() -> ("Minimum"=w437:dbl)  [unwired: 2 in, 2 out]
            n186 = Multiply(x=w438, y=w445) -> (x*y=w441:dbl)
            n187 = Multiply(x=w428, y=w445) -> (x*y=w434:dbl)
            n188 = In Range and Coerce(upper limit=w443, x=w441, lower limit=w444) -> (coerced(x)=w442:dbl)  [unwired: 1 out]
            n189 = In Range and Coerce(upper limit=w436, x=w434, lower limit=w437) -> (coerced(x)=w435:dbl)  [unwired: 1 out]
            n190 = To Long Integer(number=w442) -> (32bit integer=w440:i32)
            n191 = To Long Integer(number=w435) -> (32bit integer=w431:i32)
            n192 = property on="Y Velocity SP step/sec" class="DigNum (strict)"("Val(Sgnl)"=w440) -> ()  [unwired: 2 in, 2 out]
            n193 = property on="Y Step SP" class="DigNum (strict)"("Val(Sgnl)"=w431) -> ()  [unwired: 2 in, 2 out]
          }
        }
      }
      frame #2 {
        n194 = case shown="True" "Z Jog Set" {
          frame False {
          }
          frame True {
            n195 = property on="Z offset mm" class="DigNum (strict)"() -> ("Value"=w470:dbl)  [unwired: 2 in, 2 out]
            n196 = property on="APX:FZabs" class="DigNum (strict)"() -> ("Value"=w472:dbl)  [unwired: 2 in, 2 out]
            n197 = property on="FZ Velocity SP mm/sec" class="DigNum (strict)"() -> ("Value"=w457:dbl)  [unwired: 2 in, 2 out]
            n198 = property on="APX:Fzstep" class="DigNum (strict)"() -> ("Value"=w451:dbl)  [unwired: 2 in, 2 out]
            n199 = property on="Z steps/rev" class="DigNum (strict)"() -> ("Value"=w449:u32)  [unwired: 2 in, 2 out]
            n200 = property on="Z mm/rev" class="DigNum (strict)"() -> ("Value"=w469:dbl)  [unwired: 2 in, 2 out]
            n201 = Subtract(x=w472, y=w470) -> (x-y=w471:dbl)
            n202 = Divide(x=w451, y=w469) -> (x/y=w448:dbl)
            n203 = Divide(x=w457, y=w469) -> (x/y=w456:dbl)
            n204 = Divide(x=w471, y=w469) -> (x/y=w468:dbl)
            n205 = property on="Z Velocity SP step/sec" class="DigNum (strict)"() -> ("Maximum"=w461:dbl)  [unwired: 2 in, 2 out]
            n206 = property on="Z Velocity SP step/sec" class="DigNum (strict)"() -> ("Minimum"=w462:dbl)  [unwired: 2 in, 2 out]
            n207 = To Double Precision Float(number=w449) -> (double precision float=w467:dbl)
            n208 = property on="Z Step SP" class="DigNum (strict)"() -> ("Maximum"=w454:dbl)  [unwired: 2 in, 2 out]
            n209 = property on="Z Step SP" class="DigNum (strict)"() -> ("Minimum"=w455:dbl)  [unwired: 2 in, 2 out]
            n210 = property on="Z Step SP" class="DigNum (strict)"() -> ("Maximum"=w464:dbl)  [unwired: 2 in, 2 out]
            n211 = property on="Z Step SP" class="DigNum (strict)"() -> ("Minimum"=w465:dbl)  [unwired: 2 in, 2 out]
            n212 = Multiply(x=w448, y=w467) -> (x*y=w452:dbl)
            n213 = Multiply(x=w456, y=w467) -> (x*y=w459:dbl)
            n214 = Multiply(x=w468, y=w467) -> (x*y=w466:dbl)
            n215 = In Range and Coerce(upper limit=w454, x=w452, lower limit=w455) -> (coerced(x)=w453:dbl)  [unwired: 1 out]
            n216 = In Range and Coerce(upper limit=w461, x=w459, lower limit=w462) -> (coerced(x)=w460:dbl)  [unwired: 1 out]
            n217 = In Range and Coerce(upper limit=w464, x=w466, lower limit=w465) -> (coerced(x)=w463:dbl)  [unwired: 1 out]
            n218 = To Long Integer(number=w453) -> (32bit integer=w450:i32)
            n219 = To Long Integer(number=w460) -> (32bit integer=w458:i32)
            n220 = To Long Integer(number=w463) -> ()  [unwired: 1 out]
            n221 = property on="Z Step SP" class="DigNum (strict)"("Val(Sgnl)"=w450) -> ()  [unwired: 2 in, 2 out]
            n222 = property on="Z Velocity SP step/sec" class="DigNum (strict)"("Val(Sgnl)"=w458) -> ()  [unwired: 2 in, 2 out]
          }
        }
      }
      frame #3 {
        n223 = local read "APX:FX_UP"() -> (w473:bool)
        n224 = local read "FX Jog Counts In Range?"() -> (w474:bool)
        n225 = And(x=w473, y=w474) -> (x .and. y?=w475:bool)
        n226 = case shown="True" w475 {
          tunnel: w477 -> [_ w482]
          tunnel: w476 -> [_ w481]
          frame False {
          }
          frame True {
            n227 = flat-sequence {
              tunnel: [w493] -> w488
              tunnel: [w490] -> w487
              tunnel: [w489] -> w486
              tunnel: w482 -> [w495]
              tunnel: w481 -> [w494]
              tunnel: w488 -> [w502]
              tunnel: [w501] -> w485
              tunnel: w487 -> [w503]
              tunnel: [w504] -> w484
              tunnel: w486 -> [w500]
              tunnel: [w500] -> w483
              tunnel: w485 -> [w515]
              tunnel: w484 -> [w514]
              tunnel: [w513] -> _
              tunnel: [w512] -> _
              tunnel: w483 -> [w511]
              frame #0 {
                w489 = 0.1 ("Delay Time (s)")
                n228 = property on="X Velocity SP step/sec" class="DigNum (strict)"() -> ("Value"=w492:i32)  [unwired: 2 in, 2 out]
                n229 = property on="X steps/rev" class="DigNum (strict)"() -> ("Value"=w496:u32)  [unwired: 2 in, 2 out]
                n230 = Divide(x=w492, y=w496) -> (x/y=w497:dbl)
                n231 = Number To Fractional String(number=w497) -> (F-format string=w498:string)  [unwired: 3 in]
                n232 = call "Applied Send Command.vi"("error in (no error)"=w494, "Extra"=w498, "Command"=T2."Velocity Setting", "VISA resource name"=w495) -> ("error out"=w491:errorcluster, "VISA resource name out"=w493:refnum<visa-resource-name>)  [unwired: 3 in, 1 out]
                n233 = call "Time Delay14"("error in (no error)"=w491, "Delay Time (s)"=w489) -> ("error out"=w490:errorcluster)  [unwired: 9 in]
              }
              frame #1 {
                # "Distance/Position"
                n234 = property on="X Step SP" class="DigNum (strict)"() -> ("Value"=w505:i32)  [unwired: 2 in, 2 out]
                n235 = Number To Decimal String(number=w505) -> (decimal integer string=w507:string)  [unwired: 1 in]
                n236 = call "Applied Send Command.vi"("error in (no error)"=w503, "Extra"=w507, "Command"=T2."Distance or Position", "VISA resource name"=w502) -> ("error out"=w506:errorcluster, "VISA resource name out"=w501:refnum<visa-resource-name>)  [unwired: 3 in, 1 out]
                n237 = call "Time Delay31"("error in (no error)"=w506, "Delay Time (s)"=w500) -> ("error out"=w504:errorcluster)  [unwired: 9 in]
              }
              frame #2 {
                # "Feed to Position"
                n238 = call "Applied Send Command.vi"("error in (no error)"=w514, "Command"=T2."Feed to Length", "VISA resource name"=w515) -> ("error out"=w509:errorcluster, "VISA resource name out"=w513:refnum<visa-resource-name>)  [unwired: 4 in, 1 out]
                n239 = call "Time Delay15"("error in (no error)"=w509, "Delay Time (s)"=w511) -> ("error out"=w512:errorcluster)  [unwired: 9 in]
              }
            }
            n240 = local read "FX Jog counts"() -> (w480:i8)
            n241 = Increment(x=w480) -> (x+1=w479:i8)
            n242 = local write "FX Jog counts"(w479) -> ()
            n243 = local write "APX:FX_UP"(FALSE ("Jog X+")) -> ()
          }
        }
      }
      frame #4 {
        n244 = local read "APX:FX_DOWN"() -> (w516:bool)
        n245 = local read "FX Jog Counts In Range?"() -> (w517:bool)
        n246 = And(x=w516, y=w517) -> (x .and. y?=w518:bool)
        n247 = case shown="True" w518 {
          tunnel: w520 -> [_ w525]
          tunnel: w519 -> [_ w524]
          frame False {
          }
          frame True {
            n248 = local read "FX Jog counts"() -> (w523:i8)
            n249 = flat-sequence {
              tunnel: [w538] -> w531
              tunnel: [w535] -> w530
              tunnel: [w534] -> w529
              tunnel: [w533] -> _
              tunnel: w525 -> [w533]
              tunnel: w524 -> [w532]
              tunnel: w531 -> [w547]
              tunnel: [w546] -> w528
              tunnel: w530 -> [w548]
              tunnel: [w549] -> w527
              tunnel: w529 -> [w545]
              tunnel: [w545] -> w526
              tunnel: w528 -> [w560]
              tunnel: w527 -> [w559]
              tunnel: [w558] -> _
              tunnel: [w557] -> _
              tunnel: w526 -> [w556]
              frame #0 {
                w534 = 0.1 ("Delay Time (s)")
                n250 = property on="X Velocity SP step/sec" class="DigNum (strict)"() -> ("Value"=w537:i32)  [unwired: 2 in, 2 out]
                n251 = property on="X steps/rev" class="DigNum (strict)"() -> ("Value"=w539:u32)  [unwired: 2 in, 2 out]
                n252 = Divide(x=w537, y=w539) -> (x/y=w540:dbl)
                n253 = Number To Fractional String(number=w540) -> (F-format string=w541:string)  [unwired: 3 in]
                n254 = call "Applied Send Command.vi"("error in (no error)"=w532, "Extra"=w541, "Command"=T2."Velocity Setting", "VISA resource name"=w533) -> ("error out"=w536:errorcluster, "VISA resource name out"=w538:refnum<visa-resource-name>)  [unwired: 3 in, 1 out]
                n255 = call "Time Delay6"("error in (no error)"=w536, "Delay Time (s)"=w534) -> ("error out"=w535:errorcluster)  [unwired: 9 in]
              }
              frame #1 {
                # "Distance/Position"
                n256 = property on="X Step SP" class="DigNum (strict)"() -> ("Value"=w550:i32)  [unwired: 2 in, 2 out]
                n257 = Multiply(x=-1, y=w550) -> (x*y=w544:i32)
                n258 = Number To Decimal String(number=w544) -> (decimal integer string=w552:string)  [unwired: 1 in]
                n259 = call "Applied Send Command.vi"("error in (no error)"=w548, "Extra"=w552, "Command"=T2."Distance or Position", "VISA resource name"=w547) -> ("error out"=w551:errorcluster, "VISA resource name out"=w546:refnum<visa-resource-name>)  [unwired: 3 in, 1 out]
                n260 = call "Time Delay7"("error in (no error)"=w551, "Delay Time (s)"=w545) -> ("error out"=w549:errorcluster)  [unwired: 9 in]
              }
              frame #2 {
                # "Feed to Position"
                n261 = call "Applied Send Command.vi"("error in (no error)"=w559, "Command"=T2."Feed to Length", "VISA resource name"=w560) -> ("error out"=w554:errorcluster, "VISA resource name out"=w558:refnum<visa-resource-name>)  [unwired: 4 in, 1 out]
                n262 = call "Time Delay5"("error in (no error)"=w554, "Delay Time (s)"=w556) -> ("error out"=w557:errorcluster)  [unwired: 9 in]
              }
            }
            n263 = Decrement(x=w523) -> (x-1=w522:i8)
            n264 = local write "FX Jog counts"(w522) -> ()
            n265 = local write "APX:FX_DOWN"(FALSE ("Jog X-")) -> ()
          }
        }
      }
      frame #5 {
        n266 = local read "FY Jog Counts In Range?"() -> (w562:bool)
        n267 = local read "APX:FY_UP"() -> (w561:bool)
        n268 = And(x=w562, y=w561) -> (x .and. y?=w563:bool)
        n269 = case shown="True" w563 {
          tunnel: w565 -> [_ w570]
          tunnel: w564 -> [_ w569]
          frame False {
          }
          frame True {
            n270 = local read "FY Jog counts"() -> (w568:i8)
            n271 = local write "APX:FY_UP"(FALSE ("Jog Y+")) -> ()
            n272 = Increment(x=w568) -> (x+1=w567:i8)
            n273 = local write "FY Jog counts"(w567) -> ()
            n274 = flat-sequence {
              tunnel: [w583] -> w576
              tunnel: [w578] -> w575
              tunnel: [w577] -> w574
              tunnel: w569 -> [w582]
              tunnel: w570 -> [w581]
              tunnel: [w594] -> w573
              tunnel: [w589] -> w572
              tunnel: w576 -> [w592]
              tunnel: w575 -> [w593]
              tunnel: w574 -> [w590]
              tunnel: [w590] -> w571
              tunnel: [w599] -> _
              tunnel: [w602] -> _
              tunnel: w573 -> [w601]
              tunnel: w572 -> [w600]
              tunnel: w571 -> [w603]
              frame #0 {
                w577 = 0.5 ("Delay Time (s)")
                # "Velocity Setting"
                n275 = property on="Y Velocity SP step/sec" class="DigNum (strict)"() -> ("Value"=w586:i32)  [unwired: 2 in, 2 out]
                n276 = property on="Y steps/rev" class="DigNum (strict)"() -> ("Value"=w585:u32)  [unwired: 2 in, 2 out]
                n277 = Number To Decimal String(number=w586) -> ()  [unwired: 1 in, 1 out]
                n278 = Divide(x=w586, y=w585) -> (x/y=w587:dbl)
                n279 = Number To Fractional String(number=w587) -> (F-format string=w580:string)  [unwired: 3 in]
                n280 = call "Applied Send Command.vi"("error in (no error)"=w582, "Extra"=w580, "Command"=T2."Velocity Setting", "VISA resource name"=w581) -> ("error out"=w579:errorcluster, "VISA resource name out"=w583:refnum<visa-resource-name>)  [unwired: 3 in, 1 out]
                n281 = call "Time Delay22"("error in (no error)"=w579, "Delay Time (s)"=w577) -> ("error out"=w578:errorcluster)  [unwired: 9 in]
              }
              frame #1 {
                # "Move to Abs Position"
                n282 = property on="Y Step SP" class="DigNum (strict)"() -> ("Value"=w596:i32)  [unwired: 2 in, 2 out]
                n283 = Number To Decimal String(number=w596) -> (decimal integer string=w591:string)  [unwired: 1 in]
                n284 = call "Applied Send Command.vi"("error in (no error)"=w593, "Extra"=w591, "Command"=T2."Distance or Position", "VISA resource name"=w592) -> ("error out"=w588:errorcluster, "VISA resource name out"=w594:refnum<visa-resource-name>)  [unwired: 3 in, 1 out]
                n285 = call "Time Delay"("error in (no error)"=w588, "Delay Time (s)"=w590) -> ("error out"=w589:errorcluster)  [unwired: 9 in]
              }
              frame #2 {
                n286 = call "Applied Send Command.vi"("error in (no error)"=w600, "Command"=T2."Feed to Length", "VISA resource name"=w601) -> ("error out"=w597:errorcluster, "VISA resource name out"=w602:refnum<visa-resource-name>)  [unwired: 4 in, 1 out]
                n287 = call "Time Delay23"("error in (no error)"=w597, "Delay Time (s)"=w603) -> ("error out"=w599:errorcluster)  [unwired: 9 in]
              }
            }
          }
        }
      }
      frame #6 {
        n288 = local read "APX:FY_DOWN"() -> (w604:bool)
        n289 = local read "FY Jog Counts In Range?"() -> (w605:bool)
        n290 = And(x=w604, y=w605) -> (x .and. y?=w606:bool)
        n291 = case shown="True" w606 {
          tunnel: w608 -> [_ w613]
          tunnel: w607 -> [_ w612]
          frame False {
          }
          frame True {
            n292 = local read "FY Jog counts"() -> (w611:i8)
            n293 = flat-sequence {
              tunnel: [w626] -> w619
              tunnel: [w621] -> w618
              tunnel: [w620] -> w617
              tunnel: w612 -> [w625]
              tunnel: w613 -> [w624]
              tunnel: [w639] -> w616
              tunnel: [w634] -> w615
              tunnel: w619 -> [w637]
              tunnel: w618 -> [w638]
              tunnel: w617 -> [w635]
              tunnel: [w635] -> w614
              tunnel: [w644] -> _
              tunnel: [w647] -> _
              tunnel: w616 -> [w646]
              tunnel: w615 -> [w645]
              tunnel: w614 -> [w648]
              frame #0 {
                w620 = 0.5 ("Delay Time (s)")
                # "Velocity Setting"
                n294 = property on="Y Velocity SP step/sec" class="DigNum (strict)"() -> ("Value"=w629:i32)  [unwired: 2 in, 2 out]
                n295 = property on="Y steps/rev" class="DigNum (strict)"() -> ("Value"=w628:u32)  [unwired: 2 in, 2 out]
                n296 = Number To Decimal String(number=w629) -> ()  [unwired: 1 in, 1 out]
                n297 = Divide(x=w629, y=w628) -> (x/y=w630:dbl)
                n298 = Number To Fractional String(number=w630) -> (F-format string=w623:string)  [unwired: 3 in]
                n299 = call "Applied Send Command.vi"("error in (no error)"=w625, "Extra"=w623, "Command"=T2."Velocity Setting", "VISA resource name"=w624) -> ("error out"=w622:errorcluster, "VISA resource name out"=w626:refnum<visa-resource-name>)  [unwired: 3 in, 1 out]
                n300 = call "Time Delay18"("error in (no error)"=w622, "Delay Time (s)"=w620) -> ("error out"=w621:errorcluster)  [unwired: 9 in]
              }
              frame #1 {
                # "Move to Abs Position"
                n301 = property on="Y Step SP" class="DigNum (strict)"() -> ("Value"=w641:i32)  [unwired: 2 in, 2 out]
                n302 = Multiply(x=-1, y=w641) -> (x*y=w632:i32)
                n303 = Number To Decimal String(number=w632) -> (decimal integer string=w636:string)  [unwired: 1 in]
                n304 = call "Applied Send Command.vi"("error in (no error)"=w638, "Extra"=w636, "Command"=T2."Distance or Position", "VISA resource name"=w637) -> ("error out"=w633:errorcluster, "VISA resource name out"=w639:refnum<visa-resource-name>)  [unwired: 3 in, 1 out]
                n305 = call "Time Delay10"("error in (no error)"=w633, "Delay Time (s)"=w635) -> ("error out"=w634:errorcluster)  [unwired: 9 in]
              }
              frame #2 {
                n306 = call "Applied Send Command.vi"("error in (no error)"=w645, "Command"=T2."Feed to Length", "VISA resource name"=w646) -> ("error out"=w642:errorcluster, "VISA resource name out"=w647:refnum<visa-resource-name>)  [unwired: 4 in, 1 out]
                n307 = call "Time Delay9"("error in (no error)"=w642, "Delay Time (s)"=w648) -> ("error out"=w644:errorcluster)  [unwired: 9 in]
              }
            }
            n308 = Decrement(x=w611) -> (x-1=w610:i8)
            n309 = local write "FY Jog counts"(w610) -> ()
            n310 = local write "APX:FY_DOWN"(FALSE ("Jog Y-")) -> ()
          }
        }
      }
      frame #7 {
        n311 = local read "FZ Jog Counts In Range?"() -> (w650:bool)
        n312 = local read "APX:FZ_UP"() -> (w649:bool)
        n313 = And(x=w649, y=w650) -> (x .and. y?=w651:bool)
        n314 = case shown="True" w651 {
          tunnel: w653 -> [_ w658]
          tunnel: w652 -> [_ w657]
          frame False {
          }
          frame True {
            n315 = local read "FZ Jog counts"() -> (w656:i8)
            n316 = flat-sequence {
              tunnel: [w670] -> w664
              tunnel: [w668] -> w663
              tunnel: [w667] -> w662
              tunnel: w658 -> [w666]
              tunnel: w657 -> [w665]
              tunnel: [w679] -> w661
              tunnel: [w678] -> w660
              tunnel: w664 -> [w680]
              tunnel: w663 -> [w682]
              tunnel: w662 -> [w676]
              tunnel: [w676] -> w659
              tunnel: [w691] -> _
              tunnel: [w688] -> _
              tunnel: w661 -> [w689]
              tunnel: w660 -> [w687]
              tunnel: w659 -> [w690]
              frame #0 {
                w667 = 0.1 ("Delay Time (s)")
                n317 = property on="Z Velocity SP step/sec" class="DigNum (strict)"() -> ("Value"=w672:i32)  [unwired: 2 in, 2 out]
                n318 = property on="Z steps/rev" class="DigNum (strict)"() -> ("Value"=w671:u32)  [unwired: 2 in, 2 out]
                n319 = Divide(x=w672, y=w671) -> (x/y=w673:dbl)
                n320 = Number To Fractional String(number=w673) -> (F-format string=w674:string)  [unwired: 3 in]
                n321 = call "Applied Send Command.vi"("error in (no error)"=w665, "Extra"=w674, "Command"=T2."Velocity Setting", "VISA resource name"=w666) -> ("error out"=w669:errorcluster, "VISA resource name out"=w670:refnum<visa-resource-name>)  [unwired: 3 in, 1 out]
                n322 = call "Time Delay52"("error in (no error)"=w669, "Delay Time (s)"=w667) -> ("error out"=w668:errorcluster)  [unwired: 9 in]
              }
              frame #1 {
                # "Move to Abs Position"
                n323 = property on="Z Step SP" class="DigNum (strict)"() -> ("Value"=w684:i32)  [unwired: 2 in, 2 out]
                n324 = Number To Decimal String(number=w684) -> (decimal integer string=w681:string)  [unwired: 1 in]
                n325 = call "Applied Send Command.vi"("error in (no error)"=w682, "Extra"=w681, "Command"=T2."Distance or Position", "VISA resource name"=w680) -> ("error out"=w677:errorcluster, "VISA resource name out"=w679:refnum<visa-resource-name>)  [unwired: 3 in, 1 out]
                n326 = call "Time Delay51"("error in (no error)"=w677, "Delay Time (s)"=w676) -> ("error out"=w678:errorcluster)  [unwired: 9 in]
              }
              frame #2 {
                n327 = call "Applied Send Command.vi"("error in (no error)"=w687, "Command"=T2."Feed to Length", "VISA resource name"=w689) -> ("error out"=w685:errorcluster, "VISA resource name out"=w688:refnum<visa-resource-name>)  [unwired: 4 in, 1 out]
                n328 = call "Time Delay28"("error in (no error)"=w685, "Delay Time (s)"=w690) -> ("error out"=w691:errorcluster)  [unwired: 9 in]
              }
            }
            n329 = Increment(x=w656) -> (x+1=w655:i8)
            n330 = local write "FZ Jog counts"(w655) -> ()
            n331 = local write "APX:FZ_UP"(FALSE ("Jog Z+")) -> ()
          }
        }
      }
      frame #8 {
        n332 = local read "APX:FZ_DOWN"() -> (w692:bool)
        n333 = local read "FZ Jog Counts In Range?"() -> (w693:bool)
        n334 = And(x=w693, y=w692) -> (x .and. y?=w694:bool)
        n335 = case shown="True" w694 {
          tunnel: w696 -> [_ w701]
          tunnel: w695 -> [_ w700]
          frame False {
          }
          frame True {
            n336 = local read "FZ Jog counts"() -> (w699:i8)
            n337 = flat-sequence {
              tunnel: [w711] -> w707
              tunnel: [w709] -> w706
              tunnel: [w708] -> w705
              tunnel: w700 -> [w712]
              tunnel: w701 -> [w713]
              tunnel: [w724] -> w704
              tunnel: [w723] -> w703
              tunnel: w707 -> [w725]
              tunnel: w706 -> [w727]
              tunnel: w705 -> [w721]
              tunnel: [w721] -> w702
              tunnel: [w736] -> _
              tunnel: [w733] -> _
              tunnel: w704 -> [w734]
              tunnel: w703 -> [w732]
              tunnel: w702 -> [w735]
              frame #0 {
                w708 = 0.1 ("Delay Time (s)")
                n338 = property on="Z Velocity SP step/sec" class="DigNum (strict)"() -> ("Value"=w715:i32)  [unwired: 2 in, 2 out]
                n339 = property on="Z steps/rev" class="DigNum (strict)"() -> ("Value"=w714:u32)  [unwired: 2 in, 2 out]
                n340 = Divide(x=w715, y=w714) -> (x/y=w716:dbl)
                n341 = Number To Fractional String(number=w716) -> (F-format string=w717:string)  [unwired: 3 in]
                n342 = call "Applied Send Command.vi"("error in (no error)"=w712, "Extra"=w717, "Command"=T2."Velocity Setting", "VISA resource name"=w713) -> ("error out"=w710:errorcluster, "VISA resource name out"=w711:refnum<visa-resource-name>)  [unwired: 3 in, 1 out]
                n343 = call "Time Delay21"("error in (no error)"=w710, "Delay Time (s)"=w708) -> ("error out"=w709:errorcluster)  [unwired: 9 in]
              }
              frame #1 {
                # "Move to Abs Position"
                n344 = property on="Z Step SP" class="DigNum (strict)"() -> ("Value"=w729:i32)  [unwired: 2 in, 2 out]
                n345 = Multiply(x=-1, y=w729) -> (x*y=w720:i32)
                n346 = Number To Decimal String(number=w720) -> (decimal integer string=w726:string)  [unwired: 1 in]
                n347 = call "Applied Send Command.vi"("error in (no error)"=w727, "Extra"=w726, "Command"=T2."Distance or Position", "VISA resource name"=w725) -> ("error out"=w722:errorcluster, "VISA resource name out"=w724:refnum<visa-resource-name>)  [unwired: 3 in, 1 out]
                n348 = call "Time Delay20"("error in (no error)"=w722, "Delay Time (s)"=w721) -> ("error out"=w723:errorcluster)  [unwired: 9 in]
              }
              frame #2 {
                n349 = call "Applied Send Command.vi"("error in (no error)"=w732, "Command"=T2."Feed to Length", "VISA resource name"=w734) -> ("error out"=w730:errorcluster, "VISA resource name out"=w733:refnum<visa-resource-name>)  [unwired: 4 in, 1 out]
                n350 = call "Time Delay19"("error in (no error)"=w730, "Delay Time (s)"=w735) -> ("error out"=w736:errorcluster)  [unwired: 9 in]
              }
            }
            n351 = Decrement(x=w699) -> (x-1=w698:i8)
            n352 = local write "FZ Jog counts"(w698) -> ()
            n353 = local write "APX:FZ_DOWN"(FALSE ("Jog Z-")) -> ()
          }
        }
      }
      frame #9 {
        n354 = local read "Move 5Z REQ"() -> (w738:bool)
        n355 = And(x=FALSE, y=w738) -> (x .and. y?=w737:bool)
        n356 = case shown="True" w737 {
          tunnel: w740 -> [_ w745]
          tunnel: w741 -> [_ w744]
          frame False {
          }
          frame True {
            n357 = flat-sequence {
              tunnel: [w757] -> w751
              tunnel: [w755] -> w750
              tunnel: [w754] -> w749
              tunnel: w745 -> [w753]
              tunnel: w744 -> [w752]
              tunnel: [w769] -> w748
              tunnel: [w768] -> w747
              tunnel: w751 -> [w770]
              tunnel: w750 -> [w772]
              tunnel: w749 -> [w766]
              tunnel: [w766] -> w746
              tunnel: [w780] -> _
              tunnel: [w777] -> _
              tunnel: w748 -> [w778]
              tunnel: w747 -> [w776]
              tunnel: w746 -> [w779]
              frame #0 {
                w754 = 0.1 ("Delay Time (s)")
                n358 = property on="Z  velocity PV step/sec" class="DigNum (strict)"() -> ("Value"=w759:i32)  [unwired: 2 in, 2 out]
                n359 = property on="Z steps/rev" class="DigNum (strict)"() -> ("Value"=w758:u32)  [unwired: 2 in, 2 out]
                n360 = Divide(x=w759, y=w758) -> (x/y=w760:dbl)
                n361 = Number To Fractional String(number=w760) -> (F-format string=w761:string)  [unwired: 3 in]
                n362 = call "Applied Send Command.vi"("error in (no error)"=w752, "Extra"=w761, "Command"=T2."Velocity Setting", "VISA resource name"=w753) -> ("error out"=w756:errorcluster, "VISA resource name out"=w757:refnum<visa-resource-name>)  [unwired: 3 in, 1 out]
                n363 = call "Time Delay24"("error in (no error)"=w756, "Delay Time (s)"=w754) -> ("error out"=w755:errorcluster)  [unwired: 9 in]
              }
              frame #1 {
                # "Move to Abs Position"
                n364 = property on="Z Step SP" class="DigNum (strict)"() -> ("Value"=w765:i32)  [unwired: 2 in, 2 out]
                n365 = Multiply(x=w765, y=1) -> (x*y=w763:i32)
                n366 = Number To Decimal String(number=w763) -> (decimal integer string=w771:string)  [unwired: 1 in]
                n367 = call "Applied Send Command.vi"("error in (no error)"=w772, "Extra"=w771, "Command"=T2."Distance or Position", "VISA resource name"=w770) -> ("error out"=w767:errorcluster, "VISA resource name out"=w769:refnum<visa-resource-name>)  [unwired: 3 in, 1 out]
                n368 = call "Time Delay25"("error in (no error)"=w767, "Delay Time (s)"=w766) -> ("error out"=w768:errorcluster)  [unwired: 9 in]
              }
              frame #2 {
                n369 = call "Applied Send Command.vi"("error in (no error)"=w776, "Command"=T2."Feed to Length", "VISA resource name"=w778) -> ("error out"=w774:errorcluster, "VISA resource name out"=w777:refnum<visa-resource-name>)  [unwired: 4 in, 1 out]
                n370 = call "Time Delay26"("error in (no error)"=w774, "Delay Time (s)"=w779) -> ("error out"=w780:errorcluster)  [unwired: 9 in]
              }
            }
            n371 = local write "FZ Jog counts"(i8 0 ("FZ Jog counts")) -> ()
            n372 = local write "Move 5Z REQ"(FALSE ("Move 5Z REQ")) -> ()
          }
        }
      }
    }
    n373 = flat-sequence {
      frame #0 {
        w313 = 0 ("index (col)")
        n374 = local read "FZ Jog Counts In Range?"() -> (w320:bool)
        n375 = local read "FX Jog Counts In Range?"() -> (w321:bool)
        n376 = local read "FY Jog Counts In Range?"() -> (w322:bool)
        n377 = local read "Z in Motion"() -> (w344:bool)
        n378 = Build Array("APX:FX_UP", "APX:FX_DOWN", "APX:FY_UP", "APX:FY_DOWN", "APX:FZ_UP", "APX:FZ_DOWN", "APX:MZ_CHK") -> (w383:string[])
        n379 = local read "X  in Motion"() -> (w346:bool)
        n380 = local read "Y in Motion"() -> (w345:bool)
        n381 = call-poly "CaLabGet.vi"("PV Names"=w383) -> ("Value Array (number)"=w311:dbl[][], "Error out"=w348:errorcluster)  [unwired: 8 in, 5 out]
        n382 = Build Array(w346, w345, w344) -> (w343:bool[])
        n383 = Or Array Elements(Boolean array=w343) -> (logical OR=w316:bool)
        "Busy" <- w316
        n384 = Build Array(w322, w321, w320) -> (w319:bool[])
        n385 = And Array Elements(Boolean array=w319) -> (logical AND=w318:bool)
        n386 = Not(x=w318) -> (.not. x?=w317:bool)
        n387 = Build Array(FALSE, w316, w317) -> (w349:bool[])
        n388 = Boolean Array To Number(Boolean array=w349) -> (number=w342:u32)
        "status" <- w342
        n389 = Build Array(w342, w342, w342, w342, w342, w342) -> (w382:u32[])
        n390 = Index Array(array=w311, index (row)=6, index (col)=w313) -> (element=w310:dbl)
        n391 = Index Array(array=w311, index (row)=0 ("disabled index (row)"), index (col)=w313) -> (element=w341:dbl)
        n392 = Index Array(array=w311, index (row)=1, index (col)=w313) -> (element=w339:dbl)
        n393 = Index Array(array=w311, index (row)=4, index (col)=w313) -> (element=w334:dbl)
        n394 = Index Array(array=w311, index (row)=2, index (col)=w313) -> (element=w338:dbl)
        n395 = Index Array(array=w311, index (row)=5, index (col)=w313) -> (element=w332:dbl)
        n396 = Index Array(array=w311, index (row)=3, index (col)=w313) -> (element=w336:dbl)
        n397 = To Unsigned Byte Integer(number=w341) -> (unsigned 8bit integer=w340:u8)
        "APX:FX_UP" <- w340
        n398 = To Unsigned Byte Integer(number=w310) -> (unsigned 8bit integer=w309:u8)
        n399 = To Unsigned Byte Integer(number=w339) -> (unsigned 8bit integer=w323:u8)
        "APX:FX_DOWN" <- w323
        n400 = To Unsigned Byte Integer(number=w334) -> (unsigned 8bit integer=w333:u8)
        "APX:FZ_UP" <- w333
        n401 = To Unsigned Byte Integer(number=w338) -> (unsigned 8bit integer=w337:u8)
        "APX:FY_UP" <- w337
        n402 = To Unsigned Byte Integer(number=w332) -> (unsigned 8bit integer=w331:u8)
        "APX:FZ_DOWN" <- w331
        "element 7" <- w331
        n403 = To Unsigned Byte Integer(number=w336) -> (unsigned 8bit integer=w335:u8)
        "APX:FY_DOWN" <- w335
        n404 = Number To Boolean Array(number=w340) -> (Boolean array=w369:bool[])
        n405 = Number To Boolean Array(number=w309) -> (Boolean array=w308:bool[])
        n406 = Number To Boolean Array(number=w323) -> (Boolean array=w367:bool[])
        n407 = Number To Boolean Array(number=w337) -> (Boolean array=w365:bool[])
        n408 = Number To Boolean Array(number=w333) -> (Boolean array=w361:bool[])
        n409 = Number To Boolean Array(number=w331) -> (Boolean array=w359:bool[])
        n410 = Number To Boolean Array(number=w335) -> (Boolean array=w363:bool[])
        n411 = Index Array(array=w369, index=0) -> (element=w355:bool)
        n412 = Index Array(array=w367, index=0) -> (element=w354:bool)
        n413 = Index Array(array=w361, index=0) -> (element=w352:bool)
        n414 = Index Array(array=w363, index=0) -> (element=w329:bool)
        n415 = Index Array(array=w365, index=0) -> (element=w353:bool)
        n416 = Index Array(array=w359, index=0) -> (element=w351:bool)
        n417 = Not(x=w316) -> (.not. x?=w315:bool)
        "x .and. y?" <- w315
        n418 = And(x=w315, y=w355) -> (x .and. y?=w324:bool)
        "element" <- w324
        n419 = And(x=w315, y=w353) -> (x .and. y?=w326:bool)
        "element 3" <- w326
        n420 = And(x=w354, y=w315) -> (x .and. y?=→"element 2":bool)
        n421 = And(x=w315, y=w352) -> (x .and. y?=w330:bool)
        "element 5" <- w330
        n422 = And(x=w315, y=w351) -> (x .and. y?=w327:bool)
        "element 6" <- w327
        n423 = disable-structure shown="Disabled" {
          disable-tunnel: w348 -> [w391 _]
          disable-tunnel: [w390 _] -> w347
          frame Enabled {
            n424 = call "Time Delay27"("error in (no error)"=w391) -> ("error out"=w390:errorcluster)  [unwired: 10 in]
          }
          frame Disabled {
          }
        }
        n425 = And(x=w315, y=w329) -> (x .and. y?=w328:bool)
        "element 4" <- w328
        n426 = call-poly <userlib>:"CaLabPut.vi"("Error in (no error)"=w347, "Values"=w382, "PV Names"=w383) -> ()  [unwired: 5 in, 4 out]
        n427 = case shown="True" "Local" {
          tunnel: [w393 "Jog Z- CNTL"] -> w375
          tunnel: [w394 "Jog Z+ CNTL"] -> w374
          tunnel: [w395 "Jog Y- CNTL"] -> w373
          tunnel: [w396 "Jog Y+ CNTL"] -> w372
          tunnel: [w397 "Jog X- CNTL"] -> w371
          tunnel: [w398 "Jog X+ CNTL"] -> w370
          tunnel: w324 -> [w398 _]
          tunnel: w354 -> [w397 _]
          tunnel: w326 -> [w396 _]
          tunnel: w328 -> [w395 _]
          tunnel: w330 -> [w394 _]
          tunnel: w327 -> [w393 _]
          tunnel: w308 -> [w392 _]
          tunnel: [w392 w399] -> w307
          frame False {
          }
          frame True {
            n428 = Build Array("APX:MZ_CHK local") -> (w399:bool[])
          }
        }
        "APX:FX_UP" <- w370
        "APX:FX_DOWN" <- w371
        "APX:FY_UP" <- w372
        "APX:FY_DOWN" <- w373
        "APX:FZ_UP" <- w374
        "APX:FZ_DOWN" <- w375
        "APX:MZ_CHK" <- w307
        "Move 5Z REQ" <- "Move 5Z"
      }
    }
    n429 = event shown="[2] \"Y Velocity SP step/sec\", \"X Velocity SP step/sec\", \"Z Velocity SP step/sec\", \"Y Step SP\", \"X Step SP\", \"Z Step SP\": Value Change" {
      selector: _ -> [_ _ _ _ _ _]
      dyn-events: _ -> [_ _ _ _ _ _]
      timeout: 1 -> [_ _ _ _ _ _]
      tunnel: w272 -> [w870 _ _ w1108 w1120 w1147]
      tunnel: [_ _ _ w1108 w1118 w1145] -> w285
      tunnel: w273 -> [w842 _ _ w1109 w1121 w1148]
      tunnel: [_ _ _ w1109 w1119 w1146] -> w284
      tunnel: w275 -> [w841 _ _ _ w1115 w1144]
      tunnel: w274 -> [w853 _ _ _ w1114 w1143]
      tunnel: [_ _ _ _ w1117 w1142] -> w282
      tunnel: [_ _ _ _ w1116 w1141] -> w281
      tunnel: w271 -> [w843 _ _ _ w1113 w1140]
      tunnel: w270 -> [w844 _ _ _ w1112 w1139]
      tunnel: [_ _ _ _ w1111 _] -> w280
      tunnel: [_ _ _ _ w1110 _] -> w279
      tunnel: [_ _ _ _ _ w1138] -> w278
      tunnel: [_ _ _ _ _ w1137] -> w277
      event Timeout {
        n430 = event-data() -> ()  [unwired: 1 in, 2 out]
        n431 = flat-sequence {
          tunnel: [w882] -> w852
          tunnel: [w895] -> w851
          tunnel: [w904] -> w850
          tunnel: [w875] -> w849
          tunnel: w843 -> [w890]
          tunnel: w844 -> [w891]
          tunnel: [w873] -> w810
          tunnel: w852 -> [w914]
          tunnel: [w914] -> w848
          tunnel: w851 -> [w913]
          tunnel: [w913] -> w847
          tunnel: w850 -> [w912]
          tunnel: [w909] -> w846
          tunnel: w849 -> [w911]
          tunnel: [w911] -> w845
          tunnel: w848 -> [w917]
          tunnel: w847 -> [w918]
          tunnel: w846 -> [w916]
          tunnel: w845 -> [w915]
          tunnel: [w915] -> w818
          frame #0 {
            w894 = 0.5 ("Delay Time (s)")
            n432 = call "Applied Send Command.vi"("error in (no error)"=w891, "Command"=T2."Immediate Position?", "VISA resource name"=w890) -> ("error out"=w889:errorcluster, "read buffer"=w886:string, "VISA resource name out"=w884:refnum<visa-resource-name>)  [unwired: 4 in]
            n433 = Hexadecimal String To Number(string=w886, offset=3) -> (number=w887:u32)  [unwired: 1 in, 1 out]
            n434 = property on="Z Step SP" class="DigNum (strict)"() -> ("Maximum"=w906:dbl)  [unwired: 2 in, 2 out]
            n435 = property on="Z Step SP" class="DigNum (strict)"() -> ("Minimum"=w908:dbl)  [unwired: 2 in, 2 out]
            n436 = To Long Integer(number=w887) -> (32bit integer=w896:i32)
            n437 = property on="Z steps/rev" class="DigNum (strict)"() -> ("Value"=w902:u32)  [unwired: 2 in, 2 out]
            n438 = property on="Z Step PV" class="DigNum (strict)"("Val(Sgnl)"=w896) -> ()  [unwired: 2 in, 2 out]
            n439 = To Long Integer(number=w906) -> (32bit integer=w905:i32)
            n440 = To Long Integer(number=w908) -> (32bit integer=w907:i32)
            n441 = In Range and Coerce(upper limit=w905, x=w896, lower limit=w907) -> (In Range?=w904:bool)  [unwired: 1 out]
            n442 = To Double Precision Float(number=w896) -> (double precision float=w897:dbl)
            n443 = To Double Precision Float(number=w902) -> (double precision float=w903:dbl)
            n444 = property on="Z in Range" class="Bool (strict)"("Val(Sgnl)"=w904) -> ()  [unwired: 2 in, 2 out]
            n445 = Divide(x=w897, y=w903) -> (x/y=w901:dbl)
            n446 = call "Time Delay17"("error in (no error)"=w889, "Delay Time (s)"=w894) -> ("error out"=w874:errorcluster)  [unwired: 9 in]
            n447 = property on="Z mm/rev" class="DigNum (strict)"() -> ("Value"=w900:dbl)  [unwired: 2 in, 2 out]
            n448 = property on="Z offset mm" class="DigNum (strict)"() -> ("Value"=w898:dbl)  [unwired: 2 in, 2 out]
            n449 = Multiply(x=w901, y=w900) -> (x*y=w899:dbl)
            n450 = call "Applied Send Command.vi"("error in (no error)"=w874, "Command"=T2."Request Status", "VISA resource name"=w884) -> ("error out"=w883:errorcluster, "read buffer"=w879:string, "VISA resource name out"=w882:refnum<visa-resource-name>)  [unwired: 4 in]
            n451 = call "Time Delay16"("error in (no error)"=w883, "Delay Time (s)"=w894) -> ("error out"=w895:errorcluster)  [unwired: 9 in]
            n452 = Add(x=w899, y=w898) -> (x+y=w873:dbl)
            n453 = String Subset(string=w879, offset (0)=0, length (rest)=1 ("length (rest)")) -> (substring=w876:string)
            n454 = property on="Z Position mm PV" class="DigNum (strict)"("Val(Sgnl)"=w873) -> ()  [unwired: 2 in, 2 out]
            n455 = Equal?(x=w876, y="R") -> (x = y?=w893:bool)
            n456 = Not Equal?(x=w876, y="R") -> (x != y?=w875:bool)
            n457 = property on="Z Ready" class="Bool (strict)"("Val(Sgnl)"=w893) -> ()  [unwired: 2 in, 2 out]
            n458 = property on="Z in Motion" class="Bool (strict)"("Val(Sgnl)"=w875) -> ()  [unwired: 2 in, 2 out]
          }
          frame #1 {
            n459 = local read "Isolated from GND?"() -> (w910:bool)
            n460 = Or(x=w910, y=w912) -> (x .or. y?=w909:bool)
          }
          frame #2 {
            n461 = case shown="False" w916 {
              tunnel: w917 -> [w922 w925]
              tunnel: [w920 w925] -> _
              tunnel: [w919 w924] -> _
              tunnel: w918 -> [w921 w924]
              frame False {
                n462 = call "Applied Send Command.vi"("error in (no error)"=w921, "Command"=T2."Stop & Kill Buffer", "VISA resource name"=w922) -> ("error out"=w919:errorcluster, "VISA resource name out"=w920:refnum<visa-resource-name>)  [unwired: 4 in, 1 out]
              }
              frame True {
              }
            }
          }
        }
        n463 = property on="Y Step SP" class="DigNum (strict)"() -> ("Maximum"=w838:dbl)  [unwired: 2 in, 2 out]
        n464 = property on="Y Step SP" class="DigNum (strict)"() -> ("Minimum"=w837:dbl)  [unwired: 2 in, 2 out]
        n465 = property on="X Step SP" class="DigNum (strict)"() -> ("Maximum"=w833:dbl)  [unwired: 2 in, 2 out]
        n466 = property on="X Step SP" class="DigNum (strict)"() -> ("Minimum"=w834:dbl)  [unwired: 2 in, 2 out]
        n467 = Subtract(x=w838, y=w837) -> (x-y=w839:dbl)
        n468 = Subtract(x=w833, y=w834) -> (x-y=w835:dbl)
        n469 = property on="X Step PV" class="DigNum (strict)"() -> ("Value"=w832:i32)  [unwired: 2 in, 2 out]
        n470 = property on="Y Step PV" class="DigNum (strict)"() -> ("Value"=w831:i32)  [unwired: 2 in, 2 out]
        n471 = Divide(x=w839, y=2.0) -> (x/y=w827:dbl)
        n472 = Divide(x=w835, y=2.0) -> (x/y=w828:dbl)
        n473 = Absolute Value(x=w832) -> (abs(x)=w829:i32)
        n474 = Absolute Value(x=w831) -> (abs(x)=w830:i32)
        n475 = Absolute Value(x=w827) -> (abs(x)=w825:dbl)
        n476 = Absolute Value(x=w828) -> (abs(x)=w826:dbl)
        n477 = Multiply(x=w829, y=w830) -> (x*y=w824:i32)
        n478 = Multiply(x=w825, y=w826) -> (x*y=w823:dbl)
        n479 = Less Or Equal?(x=w824, y=w823) -> (x <= y?=w822:bool)
        n480 = flat-sequence {
          tunnel: w870 -> [w998]
          tunnel: w842 -> [w999]
          tunnel: [w995] -> w869
          tunnel: [w1005] -> w867
          tunnel: [w984] -> w865
          tunnel: [w986] -> w863
          tunnel: w838 -> [w985]
          tunnel: w837 -> [w982]
          tunnel: w822 -> [w983]
          tunnel: [w981] -> w811
          tunnel: w869 -> [w1024]
          tunnel: [w1024] -> w868
          tunnel: w867 -> [w1023]
          tunnel: [w1023] -> w866
          tunnel: w865 -> [w1022]
          tunnel: [w1020] -> w864
          tunnel: w863 -> [w1021]
          tunnel: [w1021] -> w862
          tunnel: w868 -> [w1027]
          tunnel: w866 -> [w1028]
          tunnel: w864 -> [w1026]
          tunnel: w862 -> [w1025]
          tunnel: [w1025] -> w819
          frame #0 {
            w1004 = 0.5 ("Delay Time (s)")
            n481 = call "Applied Send Command.vi"("error in (no error)"=w998, "Command"=T2."Immediate Position?", "VISA resource name"=w999) -> ("error out"=w1001:errorcluster, "read buffer"=w1002:string, "VISA resource name out"=w996:refnum<visa-resource-name>)  [unwired: 4 in]
            n482 = To Long Integer(number=w985) -> (32bit integer=w1016:i32)
            n483 = To Long Integer(number=w982) -> (32bit integer=w1017:i32)
            n484 = Hexadecimal String To Number(string=w1002, offset=3) -> (number=w1006:u32)  [unwired: 1 in, 1 out]
            n485 = To Long Integer(number=w1006) -> (32bit integer=w1007:i32)
            n486 = property on="Y steps/rev" class="DigNum (strict)"() -> ("Value"=w1013:u32)  [unwired: 2 in, 2 out]
            n487 = property on="Y Step PV" class="DigNum (strict)"("Val(Sgnl)"=w1007) -> ()  [unwired: 2 in, 2 out]
            n488 = In Range and Coerce(upper limit=w1016, x=w1007, lower limit=w1017) -> (In Range?=w1015:bool)  [unwired: 1 out]
            n489 = To Double Precision Float(number=w1007) -> (double precision float=w1008:dbl)
            n490 = To Double Precision Float(number=w1013) -> (double precision float=w1014:dbl)
            n491 = Divide(x=w1008, y=w1014) -> (x/y=w1012:dbl)
            n492 = And(x=w1015, y=w983) -> (x .and. y?=w984:bool)
            n493 = property on="Y in Range" class="Bool (strict)"("Val(Sgnl)"=w984) -> ()  [unwired: 2 in, 2 out]
            n494 = call "Time Delay4"("error in (no error)"=w1001, "Delay Time (s)"=w1004) -> ("error out"=w994:errorcluster)  [unwired: 9 in]
            n495 = property on="Y mm/rev" class="DigNum (strict)"() -> ("Value"=w1011:dbl)  [unwired: 2 in, 2 out]
            n496 = property on="Y offset mm" class="DigNum (strict)"() -> ("Value"=w1009:dbl)  [unwired: 2 in, 2 out]
            n497 = Multiply(x=w1012, y=w1011) -> (x*y=w1010:dbl)
            n498 = call "Applied Send Command.vi"("error in (no error)"=w994, "Command"=T2."Request Status", "VISA resource name"=w996) -> ("error out"=w993:errorcluster, "read buffer"=w990:string, "VISA resource name out"=w995:refnum<visa-resource-name>)  [unwired: 4 in]
            n499 = call "Time Delay3"("error in (no error)"=w993, "Delay Time (s)"=w1004) -> ("error out"=w1005:errorcluster)  [unwired: 9 in]
            n500 = Add(x=w1010, y=w1009) -> (x+y=w981:dbl)
            n501 = String Subset(string=w990, offset (0)=0, length (rest)=1 ("length (rest)")) -> (substring=w988:string)
            n502 = property on="Y Position mm PV" class="DigNum (strict)"("Val(Sgnl)"=w981) -> ()  [unwired: 2 in, 2 out]
            n503 = Equal?(x=w988, y="R") -> (x = y?=w1003:bool)
            n504 = Not Equal?(x=w988, y="R") -> (x != y?=w986:bool)
            n505 = property on="Y Ready" class="Bool (strict)"("Val(Sgnl)"=w1003) -> ()  [unwired: 2 in, 2 out]
            n506 = property on="Y in Motion" class="Bool (strict)"("Val(Sgnl)"=w986) -> ()  [unwired: 2 in, 2 out]
          }
          frame #1 {
            n507 = local read "Isolated from GND?"() -> (w1019:bool)
            n508 = Or(x=w1022, y=w1019) -> (x .or. y?=w1020:bool)
          }
          frame #2 {
            n509 = case shown="False" w1026 {
              tunnel: w1027 -> [w1030 w1035]
              tunnel: [w1032 w1035] -> _
              tunnel: [w1031 w1034] -> _
              tunnel: w1028 -> [w1029 w1034]
              frame False {
                n510 = call "Applied Send Command.vi"("error in (no error)"=w1029, "Command"=T2."Stop & Kill Buffer", "VISA resource name"=w1030) -> ("error out"=w1031:errorcluster, "VISA resource name out"=w1032:refnum<visa-resource-name>)  [unwired: 4 in, 1 out]
              }
              frame True {
              }
            }
          }
        }
        n511 = flat-sequence {
          tunnel: [w939] -> w861
          tunnel: [w950] -> w860
          tunnel: [w928] -> w859
          tunnel: [w935] -> w858
          tunnel: w841 -> [w946]
          tunnel: w853 -> [w934]
          tunnel: w833 -> [w930]
          tunnel: w834 -> [w929]
          tunnel: w822 -> [w927]
          tunnel: [w926] -> w812
          tunnel: w861 -> [w969]
          tunnel: [w969] -> w857
          tunnel: w860 -> [w968]
          tunnel: [w968] -> w856
          tunnel: w859 -> [w965]
          tunnel: [w964] -> w855
          tunnel: w858 -> [w967]
          tunnel: [w967] -> w854
          tunnel: w857 -> [w973]
          tunnel: w856 -> [w972]
          tunnel: w855 -> [w971]
          tunnel: w854 -> [w970]
          tunnel: [w970] -> w820
          frame #0 {
            w949 = 0.5 ("Delay Time (s)")
            n512 = To Long Integer(number=w929) -> (32bit integer=w962:i32)
            n513 = To Long Integer(number=w930) -> (32bit integer=w961:i32)
            n514 = call "Applied Send Command.vi"("error in (no error)"=w934, "Command"=T2."Immediate Position?", "VISA resource name"=w946) -> ("error out"=w944:errorcluster, "read buffer"=w945:string, "VISA resource name out"=w940:refnum<visa-resource-name>)  [unwired: 4 in]
            n515 = Hexadecimal String To Number(string=w945, offset=3) -> (number=w951:u32)  [unwired: 1 in, 1 out]
            n516 = To Long Integer(number=w951) -> (32bit integer=w952:i32)
            n517 = property on="X steps/rev" class="DigNum (strict)"() -> ("Value"=w958:u32)  [unwired: 2 in, 2 out]
            n518 = property on="X Step PV" class="DigNum (strict)"("Val(Sgnl)"=w952) -> ()  [unwired: 2 in, 2 out]
            n519 = In Range and Coerce(upper limit=w961, x=w952, lower limit=w962) -> (In Range?=w960:bool)  [unwired: 1 out]
            n520 = To Double Precision Float(number=w952) -> (double precision float=w953:dbl)
            n521 = To Double Precision Float(number=w958) -> (double precision float=w959:dbl)
            n522 = Divide(x=w953, y=w959) -> (x/y=w957:dbl)
            n523 = And(x=w927, y=w960) -> (x .and. y?=w928:bool)
            n524 = property on="X  in Range" class="Bool (strict)"("Val(Sgnl)"=w928) -> ()  [unwired: 2 in, 2 out]
            n525 = call "Time Delay12"("error in (no error)"=w944, "Delay Time (s)"=w949) -> ("error out"=w937:errorcluster)  [unwired: 9 in]
            n526 = property on="X mm/rev" class="DigNum (strict)"() -> ("Value"=w956:dbl)  [unwired: 2 in, 2 out]
            n527 = property on="X offset mm" class="DigNum (strict)"() -> ("Value"=w954:dbl)  [unwired: 2 in, 2 out]
            n528 = Multiply(x=w957, y=w956) -> (x*y=w955:dbl)
            n529 = call "Applied Send Command.vi"("error in (no error)"=w937, "Command"=T2."Request Status", "VISA resource name"=w940) -> ("error out"=w938:errorcluster, "read buffer"=w942:string, "VISA resource name out"=w939:refnum<visa-resource-name>)  [unwired: 4 in]
            n530 = call "Time Delay11"("error in (no error)"=w938, "Delay Time (s)"=w949) -> ("error out"=w950:errorcluster)  [unwired: 9 in]
            n531 = Add(x=w955, y=w954) -> (x+y=w926:dbl)
            n532 = String Subset(string=w942, offset (0)=0, length (rest)=1 ("length (rest)")) -> (substring=w931:string)
            n533 = property on="X Position mm PV" class="DigNum (strict)"("Val(Sgnl)"=w926) -> ()  [unwired: 2 in, 2 out]
            n534 = Equal?(x=w931, y="R") -> (x = y?=w948:bool)
            n535 = Not Equal?(x=w931, y="R") -> (x != y?=w935:bool)
            n536 = property on="X Ready" class="Bool (strict)"("Val(Sgnl)"=w948) -> ()  [unwired: 2 in, 2 out]
            n537 = property on="X  in Motion" class="Bool (strict)"("Val(Sgnl)"=w935) -> ()  [unwired: 2 in, 2 out]
          }
          frame #1 {
            n538 = local read "Isolated from GND?"() -> (w966:bool)
            n539 = Or(x=w966, y=w965) -> (x .or. y?=w964:bool)
          }
          frame #2 {
            n540 = case shown="False" w971 {
              tunnel: w973 -> [w975 w980]
              tunnel: [w977 w980] -> _
              tunnel: [w978 w979] -> _
              tunnel: w972 -> [w974 w979]
              frame False {
                n541 = call "Applied Send Command.vi"("error in (no error)"=w974, "Command"=T2."Stop & Kill Buffer", "VISA resource name"=w975) -> ("error out"=w978:errorcluster, "VISA resource name out"=w977:refnum<visa-resource-name>)  [unwired: 4 in, 1 out]
              }
              frame True {
              }
            }
          }
        }
        n542 = Compound Arithmetic op=OR(w820, w819, w818) -> (w821:bool)
        n543 = case shown="True" w821 {
          tunnel: [T3."Enabled" ("Disabled") T3."Disabled and Grayed Out" ("Disabled")] -> w817
          frame False {
          }
          frame True {
          }
        }
        n544 = Build Array("APX:PiezoX", "APX:PiezoY", "APX:PiezoZ") -> (w816:string[])
        n545 = Build Array(w812, w811, w810) -> (w809:dbl[])
        n546 = call-poly <userlib>:"CaLabPut.vi"("Values"=w809, "PV Names"=w816) -> ()  [unwired: 6 in, 4 out]
        n547 = property on="APX:FX_DOWN" class="Bool"("DisabledEnum"=w817) -> ()  [unwired: 2 in, 2 out]
        n548 = property on="APX:FX_UP" class="Bool"("DisabledEnum"=w817) -> ()  [unwired: 2 in, 2 out]
        n549 = property on="APX:FY_UP" class="Bool"("DisabledEnum"=w817) -> ()  [unwired: 2 in, 2 out]
        n550 = property on="APX:FZ_UP" class="Bool"("DisabledEnum"=w817) -> ()  [unwired: 2 in, 2 out]
        n551 = property on="APX:FY_DOWN" class="Bool"("DisabledEnum"=w817) -> ()  [unwired: 2 in, 2 out]
        n552 = property on="APX:FZ_DOWN" class="Bool"("DisabledEnum"=w817) -> ()  [unwired: 2 in, 2 out]
      }
      event "Reset Y Position mm", "Reset X Position mm", "Reset Z Position mm": Value Change {
        n553 = event-data() -> ()  [unwired: 1 in, 5 out]
        n554 = property on="Reset Y Position mm" class="DigNum (strict)"() -> ("Value"=w1062:dbl)  [unwired: 2 in, 2 out]
        n555 = property on="Reset X Position mm" class="DigNum (strict)"() -> ("Value"=w1053:dbl)  [unwired: 2 in, 2 out]
        n556 = property on="Reset Z Position mm" class="DigNum (strict)"() -> ("Value"=w1044:dbl)  [unwired: 2 in, 2 out]
        n557 = property on="Y offset mm" class="DigNum (strict)"() -> ("Value"=w1054:dbl)  [unwired: 2 in, 2 out]
        n558 = property on="X offset mm" class="DigNum (strict)"() -> ("Value"=w1045:dbl)  [unwired: 2 in, 2 out]
        n559 = property on="Z offset mm" class="DigNum (strict)"() -> ("Value"=w1036:dbl)  [unwired: 2 in, 2 out]
        n560 = Subtract(x=w1062, y=w1054) -> (x-y=w1061:dbl)
        n561 = Subtract(x=w1053, y=w1045) -> (x-y=w1052:dbl)
        n562 = Subtract(x=w1044, y=w1036) -> (x-y=w1043:dbl)
        n563 = property on="Y steps/rev" class="DigNum (strict)"() -> ("Value"=w1056:u32)  [unwired: 2 in, 2 out]
        n564 = property on="X steps/rev" class="DigNum (strict)"() -> ("Value"=w1047:u32)  [unwired: 2 in, 2 out]
        n565 = property on="Z steps/rev" class="DigNum (strict)"() -> ("Value"=w1038:u32)  [unwired: 2 in, 2 out]
        n566 = property on="Y mm/rev" class="DigNum (strict)"() -> ("Value"=w1055:dbl)  [unwired: 2 in, 2 out]
        n567 = property on="X mm/rev" class="DigNum (strict)"() -> ("Value"=w1046:dbl)  [unwired: 2 in, 2 out]
        n568 = property on="Z mm/rev" class="DigNum (strict)"() -> ("Value"=w1037:dbl)  [unwired: 2 in, 2 out]
        n569 = Divide(x=w1061, y=w1055) -> (x/y=w1060:dbl)
        n570 = Divide(x=w1052, y=w1046) -> (x/y=w1051:dbl)
        n571 = Divide(x=w1043, y=w1037) -> (x/y=w1042:dbl)
        n572 = To Double Precision Float(number=w1056) -> (double precision float=w1059:dbl)
        n573 = To Double Precision Float(number=w1047) -> (double precision float=w1050:dbl)
        n574 = To Double Precision Float(number=w1038) -> (double precision float=w1041:dbl)
        n575 = Multiply(x=w1060, y=w1059) -> (x*y=w1058:dbl)
        n576 = Multiply(x=w1051, y=w1050) -> (x*y=w1049:dbl)
        n577 = Multiply(x=w1042, y=w1041) -> (x*y=w1040:dbl)
        n578 = To Long Integer(number=w1058) -> (32bit integer=w1057:i32)
        n579 = To Long Integer(number=w1049) -> (32bit integer=w1048:i32)
        n580 = To Long Integer(number=w1040) -> (32bit integer=w1039:i32)
        n581 = property on="Reset Y Motor Steps" class="DigNum (strict)"("Val(Sgnl)"=w1057) -> ()  [unwired: 2 in, 2 out]
        n582 = property on="Reset X Motor Steps" class="DigNum (strict)"("Val(Sgnl)"=w1048) -> ()  [unwired: 2 in, 2 out]
        n583 = property on="Reset Z Motor Steps" class="DigNum (strict)"("Val(Sgnl)"=w1039) -> ()  [unwired: 2 in, 2 out]
      }
      event "Y Velocity SP step/sec", "X Velocity SP step/sec", "Z Velocity SP step/sec", "Y Step SP", "X Step SP", "Z Step SP": Value Change {
        n584 = event-data() -> ()  [unwired: 1 in, 5 out]
        n585 = property on="X Velocity SP step/sec" class="DigNum (strict)"() -> ("Value"=w1098:i32)  [unwired: 2 in, 2 out]
        n586 = property on="Y Velocity SP step/sec" class="DigNum (strict)"() -> ("Value"=w1104:i32)  [unwired: 2 in, 2 out]
        n587 = property on="Z Velocity SP step/sec" class="DigNum (strict)"() -> ("Value"=w1092:i32)  [unwired: 2 in, 2 out]
        n588 = property on="X steps/rev" class="DigNum (strict)"() -> ("Value"=w1075:u32)  [unwired: 2 in, 2 out]
        n589 = property on="X steps/rev" class="DigNum (strict)"() -> ("Value"=w1096:u32)  [unwired: 2 in, 2 out]
        n590 = property on="Y steps/rev" class="DigNum (strict)"() -> ("Value"=w1083:u32)  [unwired: 2 in, 2 out]
        n591 = property on="Y steps/rev" class="DigNum (strict)"() -> ("Value"=w1102:u32)  [unwired: 2 in, 2 out]
        n592 = property on="Z steps/rev" class="DigNum (strict)"() -> ("Value"=w1067:u32)  [unwired: 2 in, 2 out]
        n593 = property on="Z steps/rev" class="DigNum (strict)"() -> ("Value"=w1090:u32)  [unwired: 2 in, 2 out]
        n594 = property on="X Step SP" class="DigNum (strict)"() -> ("Value"=w1077:i32)  [unwired: 2 in, 2 out]
        n595 = property on="Y Step SP" class="DigNum (strict)"() -> ("Value"=w1085:i32)  [unwired: 2 in, 2 out]
        n596 = property on="Z Step SP" class="DigNum (strict)"() -> ("Value"=w1069:i32)  [unwired: 2 in, 2 out]
        n597 = To Double Precision Float(number=w1077) -> (double precision float=w1078:dbl)
        n598 = To Double Precision Float(number=w1075) -> (double precision float=w1081:dbl)
        n599 = To Double Precision Float(number=w1098) -> (double precision float=w1099:dbl)
        n600 = To Double Precision Float(number=w1096) -> (double precision float=w1101:dbl)
        n601 = To Double Precision Float(number=w1085) -> (double precision float=w1086:dbl)
        n602 = To Double Precision Float(number=w1083) -> (double precision float=w1089:dbl)
        n603 = To Double Precision Float(number=w1104) -> (double precision float=w1105:dbl)
        n604 = To Double Precision Float(number=w1102) -> (double precision float=w1107:dbl)
        n605 = To Double Precision Float(number=w1069) -> (double precision float=w1070:dbl)
        n606 = To Double Precision Float(number=w1067) -> (double precision float=w1073:dbl)
        n607 = To Double Precision Float(number=w1092) -> (double precision float=w1093:dbl)
        n608 = To Double Precision Float(number=w1090) -> (double precision float=w1095:dbl)
        n609 = property on="X mm/rev" class="DigNum (strict)"() -> ("Value"=w1064:dbl)  [unwired: 2 in, 2 out]
        n610 = property on="Y mm/rev" class="DigNum (strict)"() -> ("Value"=w1063:dbl)  [unwired: 2 in, 2 out]
        n611 = property on="Z mm/rev" class="DigNum (strict)"() -> ("Value"=w1065:dbl)  [unwired: 2 in, 2 out]
        n612 = Divide(x=w1078, y=w1081) -> (x/y=w1080:dbl)
        n613 = Divide(x=w1099, y=w1101) -> (x/y=w1100:dbl)
        n614 = Divide(x=w1086, y=w1089) -> (x/y=w1088:dbl)
        n615 = Divide(x=w1105, y=w1107) -> (x/y=w1106:dbl)
        n616 = Divide(x=w1070, y=w1073) -> (x/y=w1072:dbl)
        n617 = Divide(x=w1093, y=w1095) -> (x/y=w1094:dbl)
        n618 = property on="X offset mm" class="DigNum (strict)"() -> ("Value"=w1074:dbl)  [unwired: 2 in, 2 out]
        n619 = property on="Y offset mm" class="DigNum (strict)"() -> ("Value"=w1082:dbl)  [unwired: 2 in, 2 out]
        n620 = property on="Z offset mm" class="DigNum (strict)"() -> ("Value"=w1066:dbl)  [unwired: 2 in, 2 out]
        n621 = Multiply(x=w1080, y=w1064) -> (x*y=w1079:dbl)
        n622 = Multiply(x=w1100, y=w1064) -> (x*y=w1097:dbl)
        n623 = Multiply(x=w1088, y=w1063) -> (x*y=w1087:dbl)
        n624 = Multiply(x=w1106, y=w1063) -> (x*y=w1103:dbl)
        n625 = Multiply(x=w1072, y=w1065) -> (x*y=w1071:dbl)
        n626 = Multiply(x=w1094, y=w1065) -> (x*y=w1091:dbl)
        n627 = property on="X Velocity MV mm/sec" class="DigNum (strict)"("Val(Sgnl)"=w1097) -> ()  [unwired: 2 in, 2 out]
        n628 = property on="Y Velocity MV mm/sec" class="DigNum (strict)"("Val(Sgnl)"=w1103) -> ()  [unwired: 2 in, 2 out]
        n629 = property on="Z Velocity MV mm/sec" class="DigNum (strict)"("Val(Sgnl)"=w1091) -> ()  [unwired: 2 in, 2 out]
        n630 = Add(x=w1079, y=w1074) -> (x+y=w1076:dbl)
        n631 = Add(x=w1087, y=w1082) -> (x+y=w1084:dbl)
        n632 = Add(x=w1071, y=w1066) -> (x+y=w1068:dbl)
        n633 = property on="X Position MV mm" class="DigNum (strict)"("Val(Sgnl)"=w1076) -> ()  [unwired: 2 in, 2 out]
        n634 = property on="Y Position MV mm" class="DigNum (strict)"("Val(Sgnl)"=w1084) -> ()  [unwired: 2 in, 2 out]
        n635 = property on="Z Position MV mm" class="DigNum (strict)"("Val(Sgnl)"=w1068) -> ()  [unwired: 2 in, 2 out]
      }
      event Application Instance Close? {
        n636 = event-data() -> ()  [unwired: 1 in, 4 out]
        n637 = event-data() -> ()  [unwired: 3 in, 1 out]
      }
      event "Stop": Mouse Down {
        n638 = event-data() -> ()  [unwired: 1 in, 7 out]
        n639 = flat-sequence {
          tunnel: [w1129] -> w1117
          tunnel: [w1128] -> w1116
          tunnel: w1115 -> [w1130]
          tunnel: w1114 -> [w1127]
          frame #0 {
            n640 = call "Applied Send Command.vi"("error in (no error)"=w1127, "Command"=T2."Stop", "VISA resource name"=w1130) -> ("error out"=w1128:errorcluster, "VISA resource name out"=w1129:refnum<visa-resource-name>)  [unwired: 4 in, 1 out]
          }
        }
        n641 = flat-sequence {
          tunnel: w1121 -> [w1133]
          tunnel: w1120 -> [w1132]
          tunnel: [w1134] -> w1119
          tunnel: [w1135] -> w1118
          frame #0 {
            n642 = call "Applied Send Command.vi"("error in (no error)"=w1132, "Command"=T2."Stop", "VISA resource name"=w1133) -> ("error out"=w1135:errorcluster, "VISA resource name out"=w1134:refnum<visa-resource-name>)  [unwired: 4 in, 1 out]
          }
        }
        n643 = flat-sequence {
          tunnel: [w1124] -> w1111
          tunnel: [w1125] -> w1110
          tunnel: w1113 -> [w1122]
          tunnel: w1112 -> [w1123]
          frame #0 {
            n644 = call "Applied Send Command.vi"("error in (no error)"=w1123, "Command"=T2."Stop", "VISA resource name"=w1122) -> ("error out"=w1125:errorcluster, "VISA resource name out"=w1124:refnum<visa-resource-name>)  [unwired: 4 in, 1 out]
          }
        }
      }
      event "Reset": Mouse Down {
        n645 = event-data() -> ()  [unwired: 1 in, 7 out]
        n646 = flat-sequence {
          tunnel: [w1156] -> w1142
          tunnel: w1143 -> [w1158]
          tunnel: [w1157] -> w1141
          tunnel: w1144 -> [w1159]
          frame #0 {
            n647 = property on="Reset X Motor Steps" class="DigNum (strict)"() -> ("Value"=w1162:i32)  [unwired: 2 in, 2 out]
            n648 = Number To Decimal String(number=w1162) -> (decimal integer string=w1160:string)  [unwired: 1 in]
            n649 = call "Applied Send Command.vi"("error in (no error)"=w1158, "Extra"=w1160, "Command"=T2."Set ABS Position", "VISA resource name"=w1159) -> ("error out"=w1157:errorcluster, "VISA resource name out"=w1156:refnum<visa-resource-name>)  [unwired: 3 in, 1 out]
          }
        }
        n650 = flat-sequence {
          tunnel: w1148 -> [w1167]
          tunnel: w1147 -> [w1164]
          tunnel: [w1166] -> w1146
          tunnel: [w1165] -> w1145
          frame #0 {
            n651 = property on="Reset Y Motor Steps" class="DigNum (strict)"() -> ("Value"=w1169:i32)  [unwired: 2 in, 2 out]
            n652 = Number To Decimal String(number=w1169) -> (decimal integer string=w1168:string)  [unwired: 1 in]
            n653 = call "Applied Send Command.vi"("error in (no error)"=w1164, "Extra"=w1168, "Command"=T2."Set ABS Position", "VISA resource name"=w1167) -> ("error out"=w1165:errorcluster, "VISA resource name out"=w1166:refnum<visa-resource-name>)  [unwired: 3 in, 1 out]
          }
        }
        n654 = flat-sequence {
          tunnel: [w1154] -> w1138
          tunnel: [w1153] -> w1137
          tunnel: w1140 -> [w1151]
          tunnel: w1139 -> [w1152]
          frame #0 {
            n655 = property on="Reset Z Motor Steps" class="DigNum (strict)"() -> ("Value"=w1155:i32)  [unwired: 2 in, 2 out]
            n656 = Number To Decimal String(number=w1155) -> (decimal integer string=w1149:string)  [unwired: 1 in]
            n657 = call "Applied Send Command.vi"("error in (no error)"=w1152, "Extra"=w1149, "Command"=T2."Set ABS Position", "VISA resource name"=w1151) -> ("error out"=w1153:errorcluster, "VISA resource name out"=w1154:refnum<visa-resource-name>)  [unwired: 3 in, 1 out]
          }
        }
      }
    }
    n658 = flat-sequence {
      frame #0 {
        w783 = 10 ("number of samples")
        n659 = local read "APX:MZ_CHK"() -> (w792:bool[])
        n660 = call "DAQ AI16"("number of samples"=w783) -> ("data"=w785:dynamicdata, "error out"=w786:errorcluster)  [unwired: 16 in, 1 out]
        n661 = call "Convert from Dynamic Data"("Dynamic Data Type"=w785) -> ("Array"=w784:dbl[])  [unwired: 3 in]
        n662 = Index Array(array=w792, index=0) -> (element=w790:bool)
        n663 = Add Array Elements(numeric array=w784) -> (sum=w782:dbl)
        n664 = Divide(x=w782, y=w783) -> (x/y=w781:dbl)
        "Io" <- w781
        n665 = Boolean To (0,1)(Boolean=w790) -> (0, 1=w797:i16)
        n666 = call "DAQ AI1"("number of samples"=w783, "error in"=w786) -> ("data"=w787:dynamicdata, "error out"=→"error out":errorcluster)  [unwired: 15 in, 1 out]
        n667 = Multiply(x=w797, y=i16 5) -> (x*y=w791:i16)
        n668 = Build Array(w790) -> (w789:bool[])
        n669 = disable-structure shown="Disabled" {
          disable-tunnel: w789 -> [w806 _]
          frame Disabled {
            n670 = call "DAQ P1.7"("data"=w806) -> ()  [unwired: 17 in, 2 out]
          }
          frame Enabled {
          }
        }
        n671 = call "Convert from Dynamic Data2"("Dynamic Data Type"=w787) -> ("Array"=w802:dbl[])  [unwired: 3 in]
        n672 = Add Array Elements(numeric array=w802) -> (sum=w801:dbl)
        n673 = Divide(x=w801, y=w783) -> (x/y=w800:dbl)
        n674 = Multiply(x=w791, y=0.8) -> (x*y=w798:dbl)
        n675 = Absolute Value(x=w800) -> (abs(x)=w795:dbl)
        "Dev1 AI1" <- w795
        n676 = Greater?(x=w795, y=w798) -> (0:w803:bool)
        n677 = call-poly <userlib>:"CaLabPut.vi"("Value"=w781, "PV Name"="BL132:Io") -> ()  [unwired: 6 in, 4 out]
        n678 = case shown="True" "Crash Override" {
          tunnel: [w807 TRUE] -> w804
          tunnel: w803 -> [w807 _]
          frame False {
          }
          frame True {
          }
        }
        "Isolated from GND?" <- w804
      }
    }
    n679 = case shown="True" "Reset Jog counts" {
      frame False {
      }
      frame True {
        w306 = 0
        n680 = local write "FY Jog counts"(w306) -> ()
        n681 = local write "FZ Jog counts"(w306) -> ()
        n682 = local write "FX Jog counts"(w306) -> ()
      }
    }
  }
  n683 = flat-sequence {
    tunnel: w37 -> [w1171]
    tunnel: w36 -> [w1170]
    tunnel: [w1182] -> w21
    frame #0 {
      # "GET CURRENT POSITION"
      n684 = call "Applied Send Command.vi"("error in (no error)"=w1170, "Extra"="", "Command"=T2."Immediate Position?", "VISA resource name"=w1171) -> ("error out"=w1172:errorcluster, "read buffer"=w1177:string, "VISA resource name out"=w1173:refnum<visa-resource-name>)  [unwired: 3 in]
      n685 = call "Applied Send Command.vi"("error in (no error)"=w1172, "Command"=T2."Stop & Kill Buffer", "VISA resource name"=w1173) -> ("error out"=w1179:errorcluster, "VISA resource name out"=w1180:refnum<visa-resource-name>)  [unwired: 4 in, 1 out]
      n686 = Hexadecimal String To Number(string=w1177, offset=3) -> (number=w1174:u32)  [unwired: 1 in, 1 out]
      n687 = VISA Close(VISA resource name=w1180, error in (no error)=w1179) -> ()  [unwired: 1 out]
      n688 = To Long Integer(number=w1174) -> (32bit integer=w1182:i32)
    }
  }
  n689 = flat-sequence {
    tunnel: w23 -> [w1185]
    tunnel: w22 -> [w1184]
    tunnel: [w1183] -> w20
    frame #0 {
      # "GET CURRENT POSITION"
      n690 = call "Applied Send Command.vi"("error in (no error)"=w1184, "Extra"="", "Command"=T2."Immediate Position?", "VISA resource name"=w1185) -> ("error out"=w1186:errorcluster, "read buffer"=w1191:string, "VISA resource name out"=w1187:refnum<visa-resource-name>)  [unwired: 3 in]
      n691 = call "Applied Send Command.vi"("error in (no error)"=w1186, "Command"=T2."Stop & Kill Buffer", "VISA resource name"=w1187) -> ("error out"=w1193:errorcluster, "VISA resource name out"=w1194:refnum<visa-resource-name>)  [unwired: 4 in, 1 out]
      n692 = Hexadecimal String To Number(string=w1191, offset=3) -> (number=w1188:u32)  [unwired: 1 in, 1 out]
      n693 = VISA Close(VISA resource name=w1194, error in (no error)=w1193) -> ()  [unwired: 1 out]
      n694 = To Long Integer(number=w1188) -> (32bit integer=w1183:i32)
    }
  }
  n695 = flat-sequence {
    tunnel: w25 -> [w1197]
    tunnel: w24 -> [w1196]
    tunnel: [w1198] -> w19
    frame #0 {
      # "GET CURRENT POSITION"
      n696 = call "Applied Send Command.vi"("error in (no error)"=w1196, "Extra"="", "Command"=T2."Immediate Position?", "VISA resource name"=w1197) -> ("error out"=w1199:errorcluster, "read buffer"=w1204:string, "VISA resource name out"=w1200:refnum<visa-resource-name>)  [unwired: 3 in]
      n697 = call "Applied Send Command.vi"("error in (no error)"=w1199, "Command"=T2."Stop & Kill Buffer", "VISA resource name"=w1200) -> ("error out"=w1206:errorcluster, "VISA resource name out"=w1207:refnum<visa-resource-name>)  [unwired: 4 in, 1 out]
      n698 = Hexadecimal String To Number(string=w1204, offset=3) -> (number=w1201:u32)  [unwired: 1 in, 1 out]
      n699 = VISA Close(VISA resource name=w1207, error in (no error)=w1206) -> ()  [unwired: 1 out]
      n700 = To Long Integer(number=w1201) -> (32bit integer=w1198:i32)
    }
  }
  n701 = flat-sequence {
    tunnel: w21 -> [w1213]
    tunnel: w20 -> [w1212]
    tunnel: w19 -> [w1211]
    frame #0 {
      n702 = Build Array(w1213, w1212, w1211) -> (w1209:i32[])
      n703 = call-poly <vilib>:"Write To Spreadsheet File.vi"("1D data"=w1209, "file path (dialog if empty)"=path "S:/SSE/SCL2/POS.TXT") -> ()  [unwired: 6 in, 1 out]
    }
    frame #1 {
    }
  }
